vi "StateMachine.vi"() -> ()   [LabVIEW 2017]
uses:
  68b3bc89-c846-434a-a9c0-588017489639.vi
panel:
  out "number as enum":enum16{"0,01%", "0,1%", "1%", "10%", "None"}(ring)
  out "DISPLAY":string
  out "unità misura":string
  in  "num/\\":bool
  in  "num_m":bool
  in  "numK":bool
  in  "numM":bool
  in  "numC":bool
  in  "numSegn":bool
  in  "num0":bool
  in  "numVirg":bool
  in  "num9":bool
  in  "num8":bool
  in  "num7":bool
  in  "num6":bool
  in  "num5":bool
  in  "num4":bool
  in  "num2":bool
  in  "num3":bool
  in  "numEnter":bool
  in  "num1":bool
  out "displayTasterino":string
  in  "SHIFT":bool
  in  "ENTER":bool
  in  "EXIT":bool
  in  "RATE":bool
  in  "DIGITS":bool
  in  "RESTR":bool
  in  "SAVE":bool
  in  "SCAN":bool
  in  "STEP":bool
  in  "RECALL":bool
  in  "STORE":bool
  in  "ON/OFF":bool
  in  "VALUE":bool
  in  "RIGHTARR":bool
  in  "LEFTARR":bool
  in  "TRIG":bool
  in  "EX TRIG":bool
  in  "RANGE DOWN":bool
  in  "AUTO":bool
  in  "RANGE UP":bool
  out "rel":string
  out "filt":string
  out "fast 0.1 PLC":string
  out "slow 5 PLC":string
  out "auto":string
  out "med 1 PLC":string
  out "CH2":string
  out "CH1":string
  in  "TEMP 2":bool
  in  "TEMP1":bool
  in  "REL":bool
  in  "FILT":bool
  in  "ACAL":bool
  in  "V1/V2":bool
  in  "DCV2":bool
  in  "DCV1":bool
  out "shift":string
  # "MX+B"
  # "%"
  # "V1 - V2"
  # "LSYNC"
  # "TYPE"
  # "OUTPUT"
  # "AOUT"
  # "TCOUPL"
  # "RANGE"
  # "SHIFT"
  # "LIMITS"
  # "BUFFER"
  # "DELAY"
  # "HOLD"
  # "RANGE"
  # "SETUP"
  # "RS232"
  # "CONFIG"
  # "HALT"
  # "GPIB"
  # "CAL"
  # "TEST"
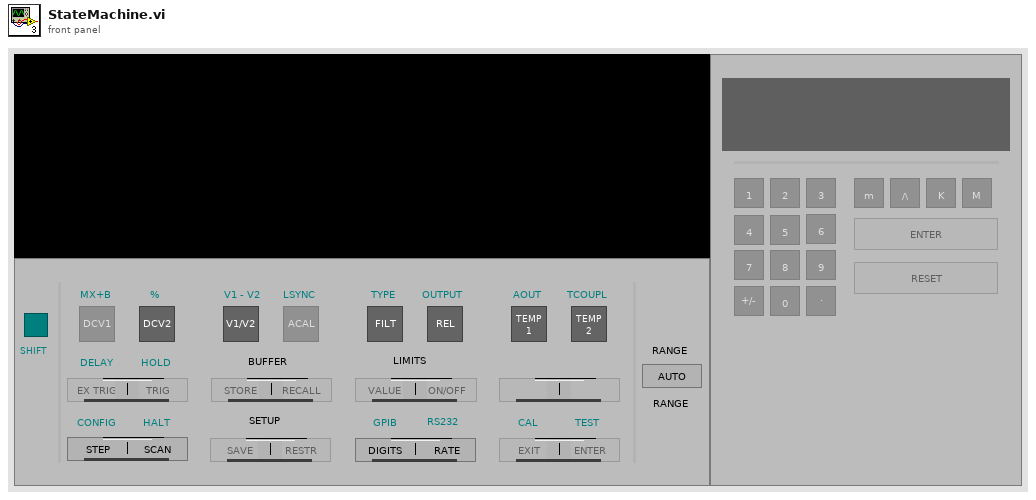
[diagram p1: front panel]
types:
  T1 = cluster{"Auto1":bool, "Auto2":bool, "Rel1":bool, "Rel2":bool, "Filt1":bool, "Filt2":bool, "Rate":enum16{"Slow", "Fast", "Med"}, "Range1":enum16{"10mV", "100mV", "1V", "10V", "100V"}, "Range2":enum16{"100mV", "1V", "10V"}, "Filt3":bool, "Filt4":bool, "Rel temp 1":bool, "Analog1":bool, "Analog2":bool, "Analog temp 1":bool, "Digital1":bool, "Digital2":bool, "Digital temp 1 ":bool, "Window1":enum16{"0,01%", "0,1%", "1%", "10%", "None"}, "Window2":enum16{"0,01%", "0,1%", "1%", "10%", "None"}, "Window temp 1":enum16{"0,01%", "0,1%", "1%", "10%", "None"}, "RDGS1":string, "RDGS2":string, "RDGS temp 1":string, "Type_type1":bool, "Type_type2":bool, "Type_type temp 1":bool, "LSync":bool, "Unit":enum16{"C", "K", "F"}, "Sens":bool, "Type tcoupl":enum16{"J", "K", "T", "E", "R", "S", "B", "N"}, "Junc":bool, "prevState":i32, "Rel temp 2":bool, "Analog temp 2":bool, "Digital temp 2":bool, "Type_type temp 2":bool, "RDGS temp 2":string, "Window temp 2":enum16{"0,01%", "0,1%", "1%", "10%", "None"}, "address":string}
  T2 = enum16{"init", "shift", "ch2", "temp1", "temp2", "v1/v2", "step", "scan", "shift_bis_volt", "v1-v2", "type_analog"}
  T3 = enum8{"Enabled", "Disabled", "Disabled and Grayed Out"}
  T4 = cluster{"Auto1":bool, "Auto2":bool, "Rel1":bool, "Rel2":bool, "Filt1":bool, "Filt2":bool, "Rate":u16, "Range1":enum16{"10mV", "100mV", "1V", "10V", "100V"}, "Range2":enum16{"100mV", "1V", "10V"}, "Filt3":bool, "Filt4":bool, "Rel temp 1":bool, "Analog1":bool, "Analog2":bool, "Analog temp 1":bool, "Digital1":bool, "Digital2":bool, "Digital temp 1 ":bool, "Window1":u16, "Window2":enum16{"0,01%", "0,1%", "1%", "10%", "None"}, "Window temp 1":enum16{"0,01%", "0,1%", "1%", "10%", "None"}, "RDGS1":string, "RDGS2":string, "RDGS temp 1":string, "Type_type1":bool, "Type_type2":bool, "Type_type temp 1":bool, "LSync":bool, "Unit":enum16{"C", "K", "F"}, "Sens":bool, "Type tcoupl":enum16{"J", "K", "T", "E", "R", "S", "B", "N"}, "Junc":bool, "prevState":i32, "Rel temp 2":bool, "Analog temp 2":bool, "Digital temp 2":bool, "Type_type temp 2":bool, "RDGS temp 2":string, "Window temp 2":enum16{"0,01%", "0,1%", "1%", "10%", "None"}, "address":string}
  T5 = cluster{"Auto1":bool, "Auto2":bool, "Rel1":bool, "Rel2":bool, "Filt1":bool, "Filt2":bool, "Rate":enum16{"Slow", "Fast", "Med"}, "Range1":enum16{"10mV", "100mV", "1V", "10V", "100V"}, "Range2":enum16{"100mV", "1V", "10V"}, "Filt3":bool, "Filt4":bool, "Rel temp 1":bool, "Analog1":bool, "Analog2":bool, "Analog temp 1":bool, "Digital1":bool, "Digital2":bool, "Digital temp 1 ":bool, "Window1":enum16{"0,01%", "0,1%", "1%", "10%", "None"}, "Window2":enum16{"0,01%", "0,1%", "1%", "10%", "None"}, "Window temp 1":enum16{"0,01%", "0,1%", "1%", "10%", "None"}, "RDGS1":string, "RDGS2":string, "RDGS temp 1":string, "Type_type1":bool, "Type_type2":bool, "Type_type temp 1":bool, "LSync":bool, "Unit":enum16{"C", "K", "F"}, "Sens":bool, "Type tcoupl":enum16{"J", "K", "T", "E", "R", "S", "B", "N"}, "Junc":bool, "prevState":i32, "Rel temp 2":bool, "Analog temp 2":bool, "Digital temp 2":bool, "Type_type temp 2":bool, "RDGS temp 2":string, "Window temp 2":enum16{"0,01%", "0,1%", "1%", "10%", "None"}, "addres":string}
  T6 = cluster{"Auto1":bool, "Auto2":bool, "Rel1":bool, "Rel2":bool, "Filt1":bool, "Filt2":bool, "Rate":enum16{"Slow", "Med", "Fast"}, "Range1":enum16{"10mV", "100mV", "1V", "10V", "100V"}, "Range2":enum16{"100mV", "1V", "10V"}, "Filt3":bool, "Filt4":bool, "Rel temp 1":bool, "Analog1":bool, "Analog2":bool, "Analog temp 1":bool, "Digital1":bool, "Digital2":bool, "Digital temp 1 ":bool, "Window1":enum16{"0,01%", "0,1%", "1%", "10%", "None"}, "Window2":enum16{"0,01%", "0,1%", "1%", "10%", "None"}, "Window temp 1":enum16{"0,01%", "0,1%", "1%", "10%", "None"}, "RDGS1":string, "RDGS2":string, "RDGS temp 1":string, "Type_type1":bool, "Type_type2":bool, "Type_type temp 1":bool, "LSync":bool, "Unit":enum16{"C", "K", "F"}, "Sens":bool, "Type tcoupl":enum16{"J", "K", "T", "E", "R", "S", "B", "N"}, "Junc":bool, "prevState":i32, "Rel temp 2":bool, "Analog temp 2":bool, "Digital temp 2":bool, "Type_type temp 2":bool, "RDGS temp 2":string, "Window temp 2":enum16{"0,01%", "0,1%", "1%", "10%", "None"}, "addres":string}
  T7 = cluster{"Auto1":bool, "Auto2":bool, "Rel1":bool, "Rel2":bool, "Filt1":bool, "Filt2":bool, "Rate":enum16{"Slow", "Med", "Fast"}, "Range1":enum16{"10mV", "100mV", "1V", "10V", "100V"}, "Range2":enum16{"100mV", "1V", "10V"}, "Filt3":bool, "Filt4":bool, "Rel temp 1":bool, "Analog1":bool, "Analog2":bool, "Analog temp 1":bool, "Digital1":bool, "Digital2":bool, "Digital temp 1 ":bool, "Window1":enum16{"0,01%", "0,1%", "1%", "10%", "None"}, "Window2":enum16{"0,01%", "0,1%", "1%", "10%", "None"}, "Window temp 1":enum16{"0,01%", "0,1%", "1%", "10%", "None"}, "RDGS1":string, "RDGS2":string, "RDGS temp 1":string, "Type_type1":bool, "Type_type2":bool, "Type_type temp 1":bool, "LSync":bool, "Unit":enum16{"C", "K", "F"}, "Sens":bool, "Type tcoupl":enum16{"J", "K", "T", "E", "R", "S", "B", "N"}, "Junc":bool, "prevState":i32, "Rel temp 2":bool, "Analog temp 2":bool, "Digital temp 2":bool, "Type_type temp 2":bool, "RDGS temp 2":string, "Window temp 2":enum16{"0,01%", "0,1%", "1%", "10%", "None"}, "address":string}
  T8 = cluster{"Auto1":bool, "Auto2":bool, "Rel1":bool, "Rel2":bool, "Filt1":bool, "Filt2":bool, "Rate":enum16{"Slow", "Fast", "Med"}, "Range1":enum16{"10mV", "100mV", "1V", "10V", "100V"}, "Range2":enum16{"100mV", "1V", "10V"}, "Filt3":bool, "Filt4":bool, "Rel temp 1":bool, "Analog1":bool, "Analog2":bool, "Analog temp 1":bool, "Digital1":bool, "Digital2":bool, "Digital temp 1 ":bool, "Window1":enum16{"None", "0,01%", "0,1%", "1%", "10%"}, "Window2":enum16{"0,01%", "0,1%", "1%", "10%", "None"}, "Window temp 1":enum16{"0,01%", "0,1%", "1%", "10%", "None"}, "RDGS1":string, "RDGS2":string, "RDGS temp 1":string, "Type_type1":bool, "Type_type2":bool, "Type_type temp 1":bool, "LSync":bool, "Unit":enum16{"C", "K", "F"}, "Sens":bool, "Type tcoupl":enum16{"J", "K", "T", "E", "R", "S", "B", "N"}, "Junc":bool, "prevState":i32, "Rel temp 2":bool, "Analog temp 2":bool, "Digital temp 2":bool, "Type_type temp 2":bool, "RDGS temp 2":string, "Window temp 2":enum16{"0,01%", "0,1%", "1%", "10%", "None"}, "address":string}
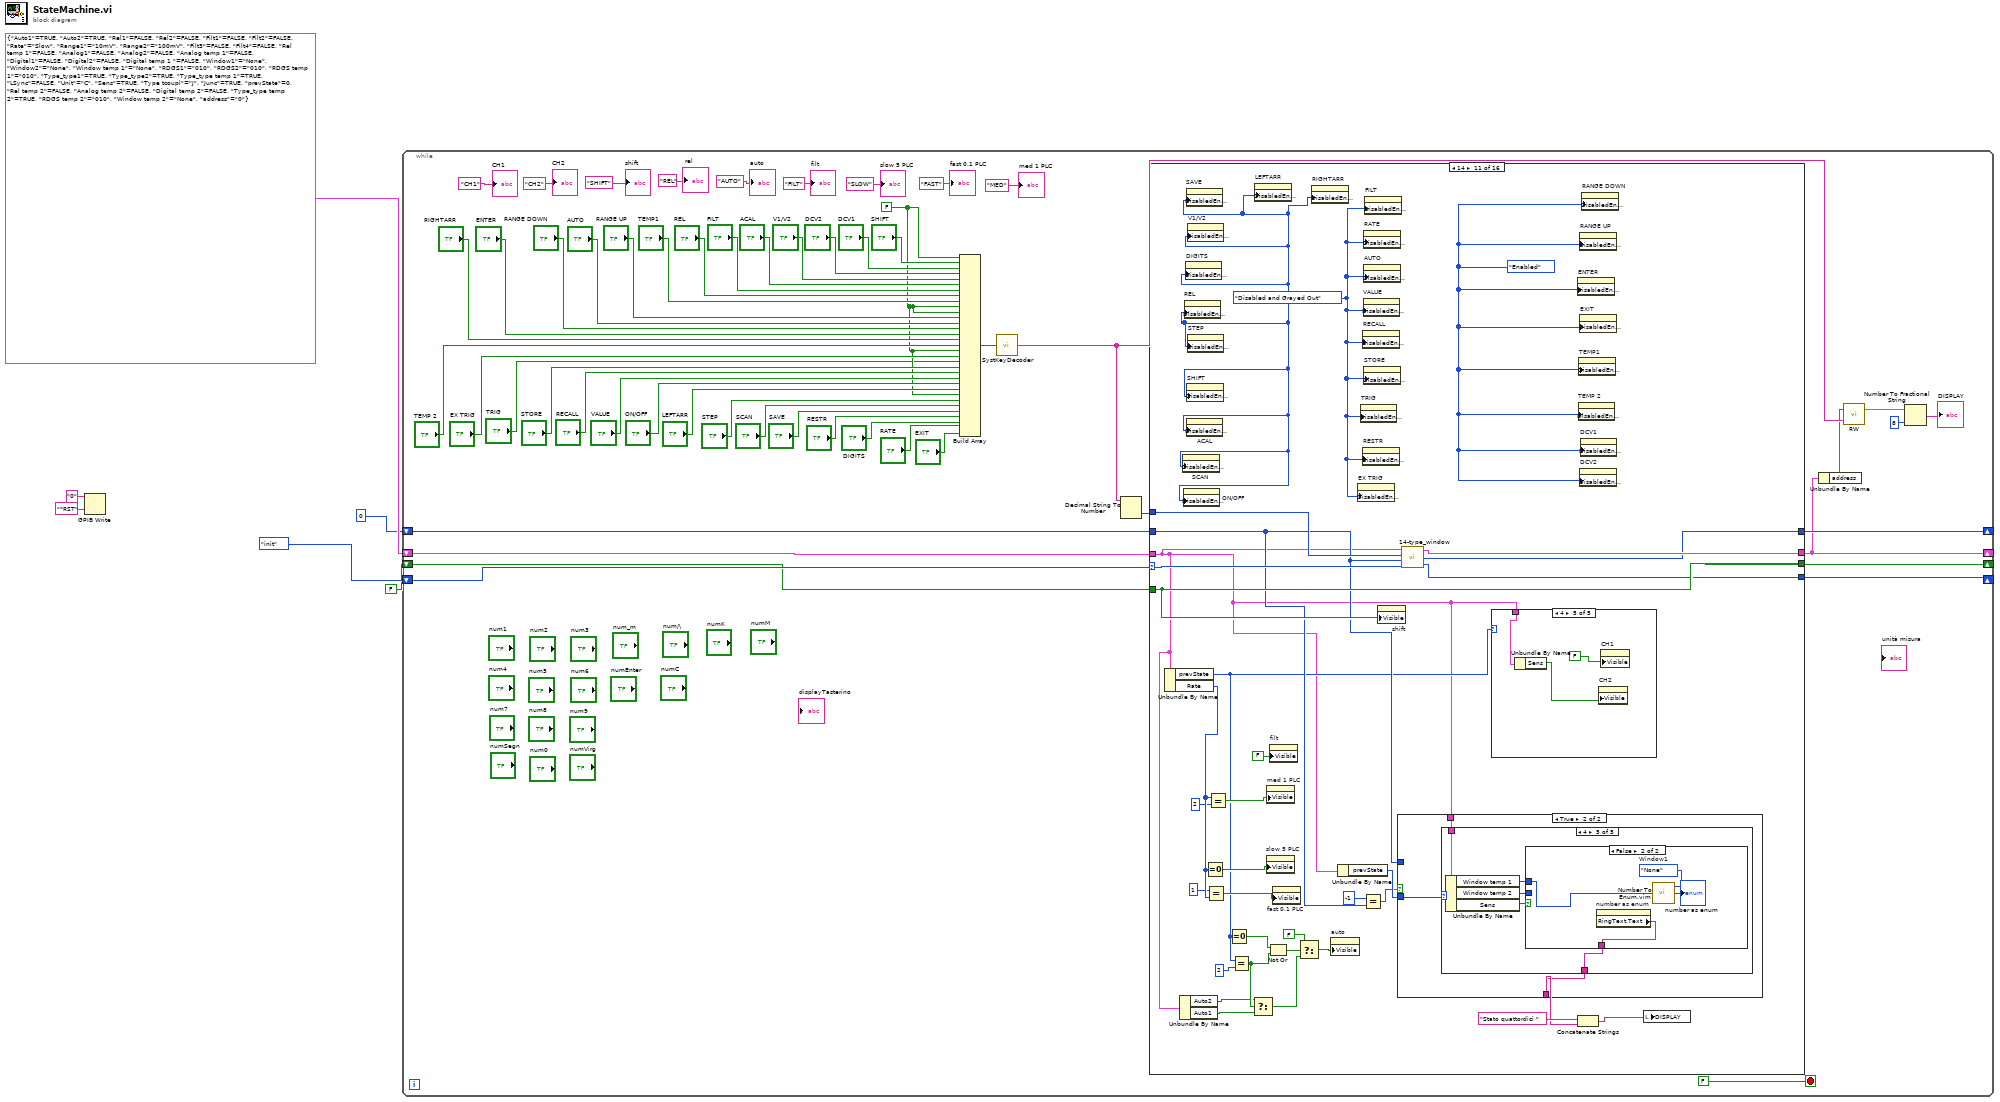
[diagram p0: block diagram]
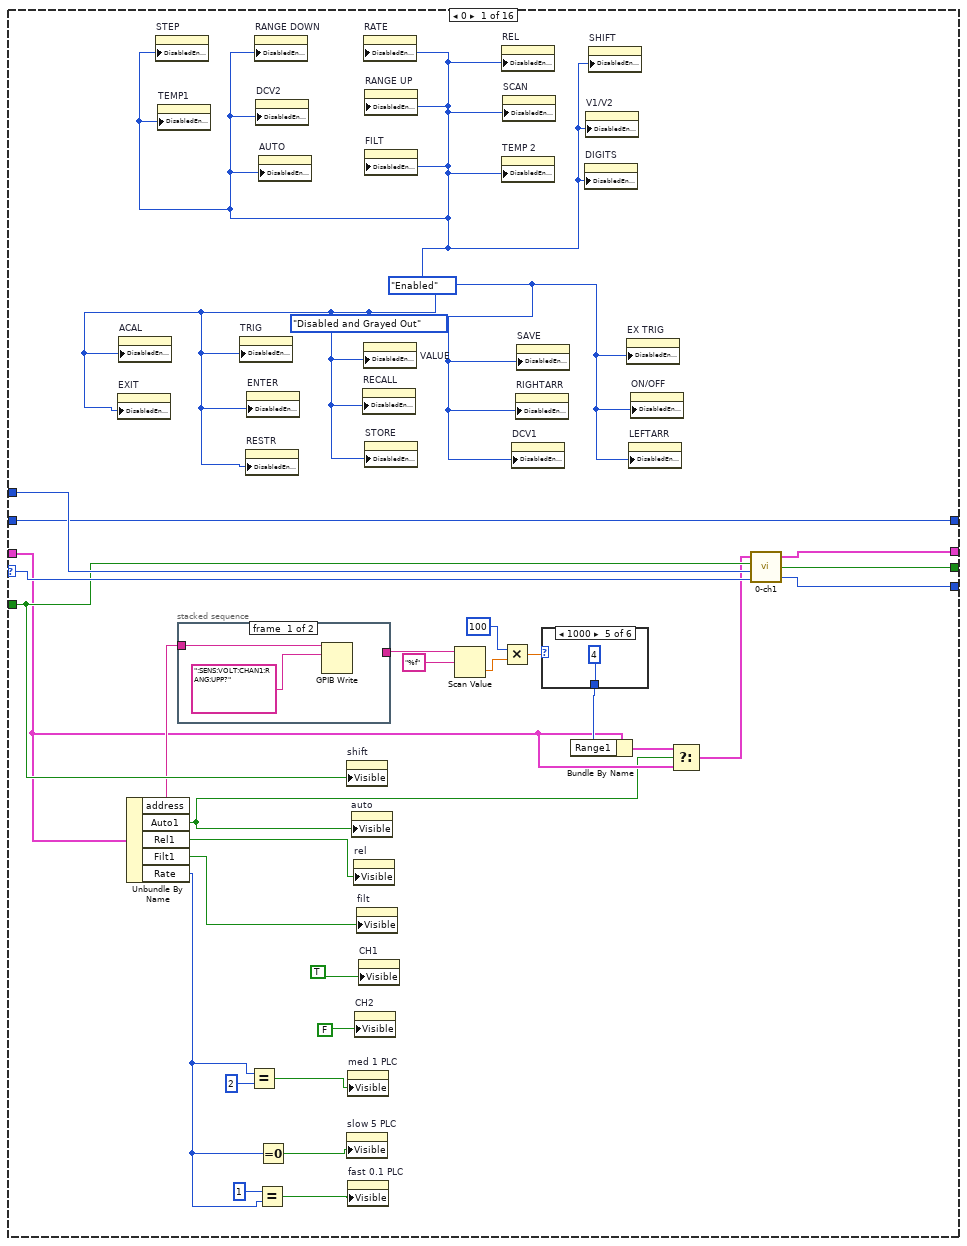
[diagram p2: hidden frame]
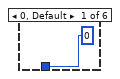
[diagram p3: hidden frame]
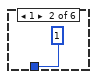
[diagram p4: hidden frame]
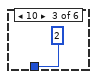
[diagram p5: hidden frame]
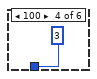
[diagram p6: hidden frame]
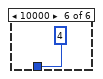
[diagram p7: hidden frame]
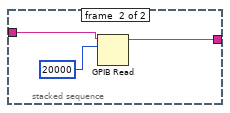
[diagram p8: hidden frame]
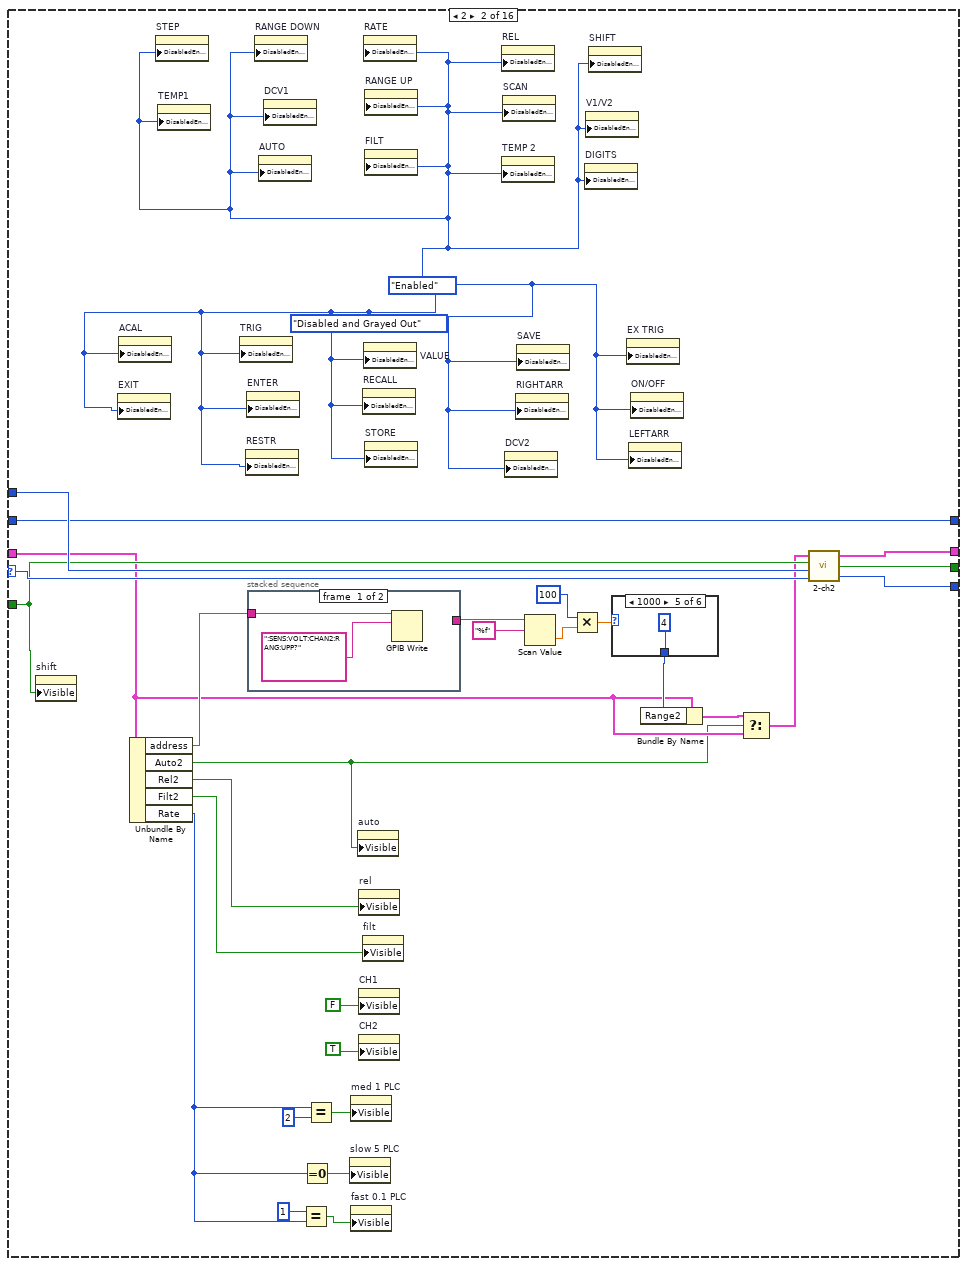
[diagram p9: hidden frame]
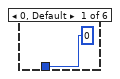
[diagram p10: hidden frame]
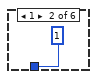
[diagram p11: hidden frame]
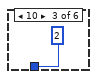
[diagram p12: hidden frame]
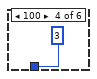
[diagram p13: hidden frame]
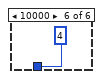
[diagram p14: hidden frame]
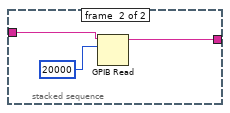
[diagram p15: hidden frame]
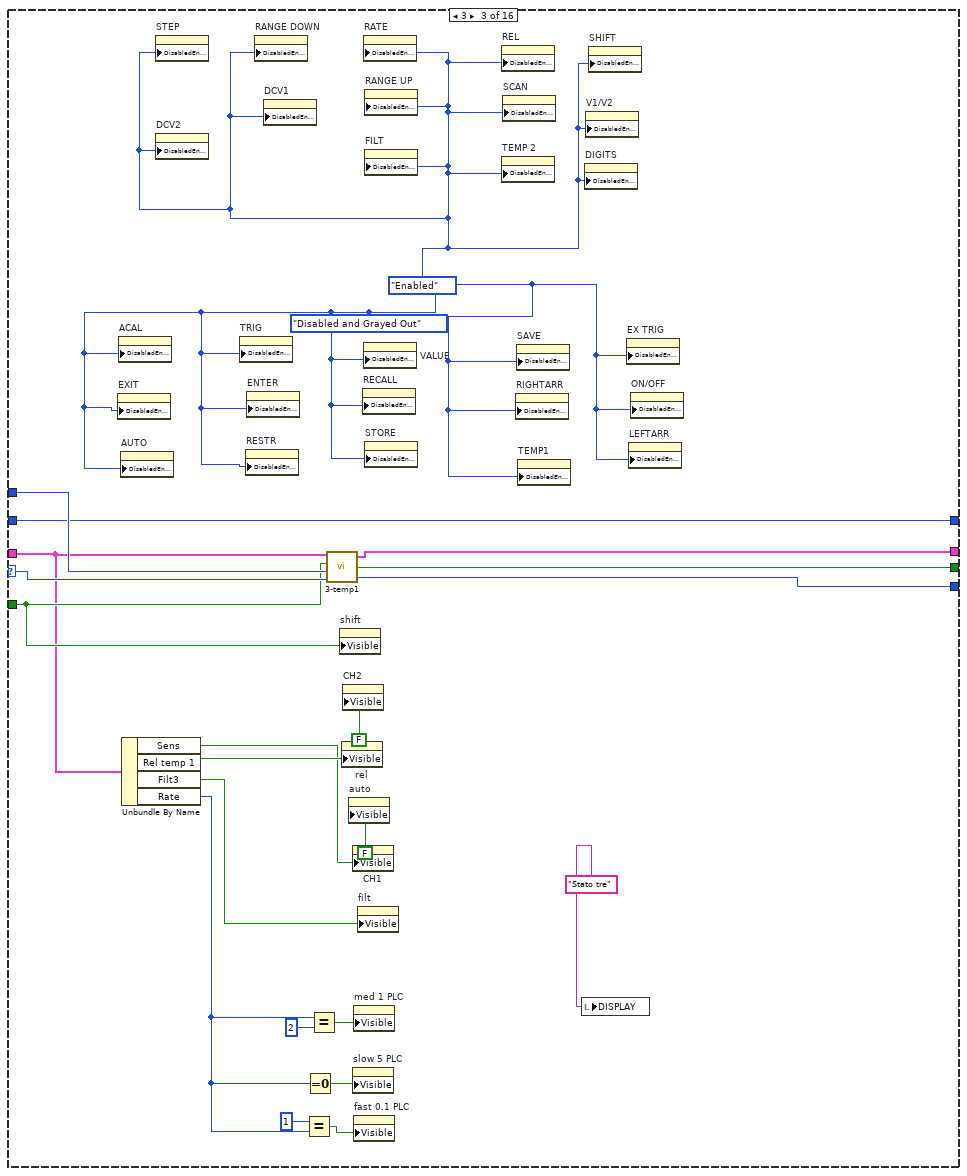
[diagram p16: hidden frame]
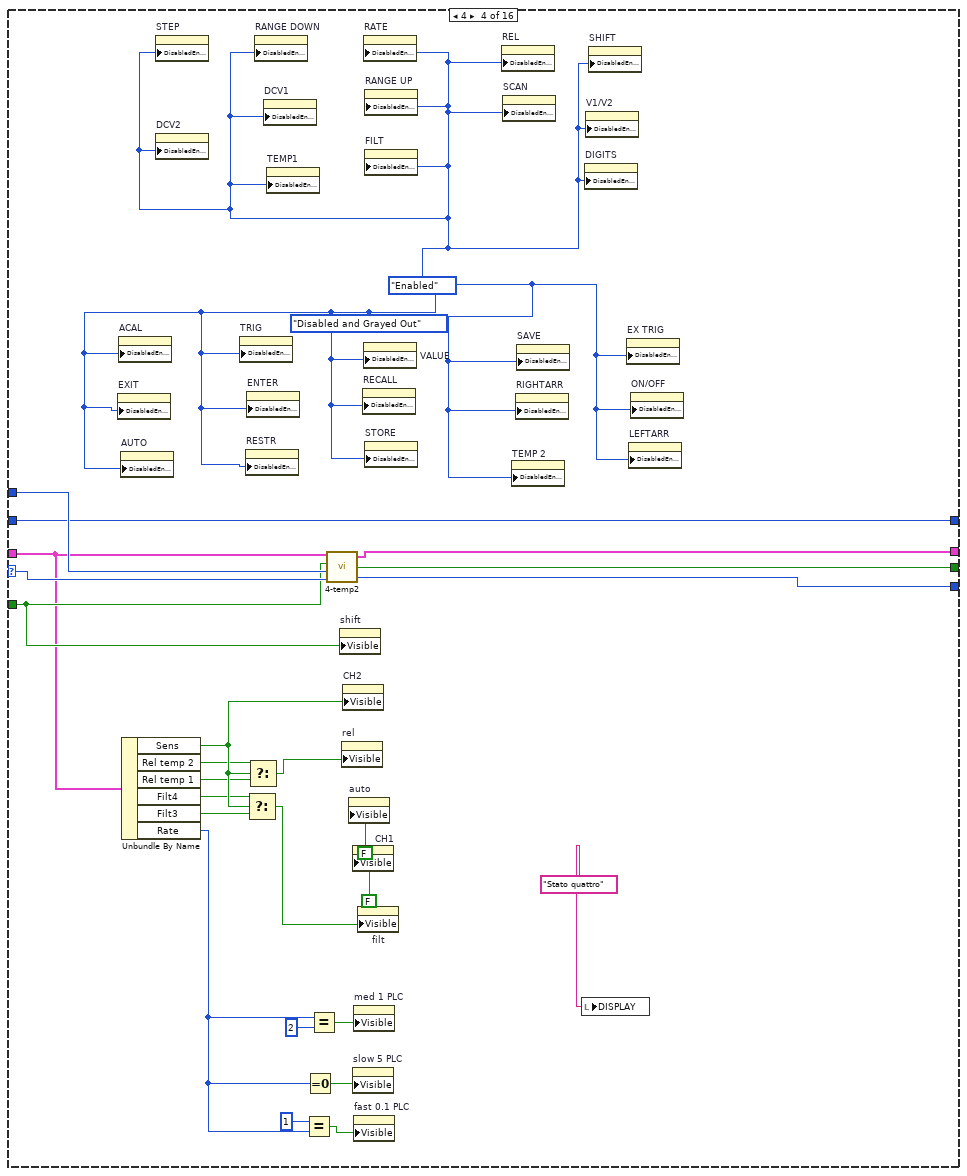
[diagram p17: hidden frame]
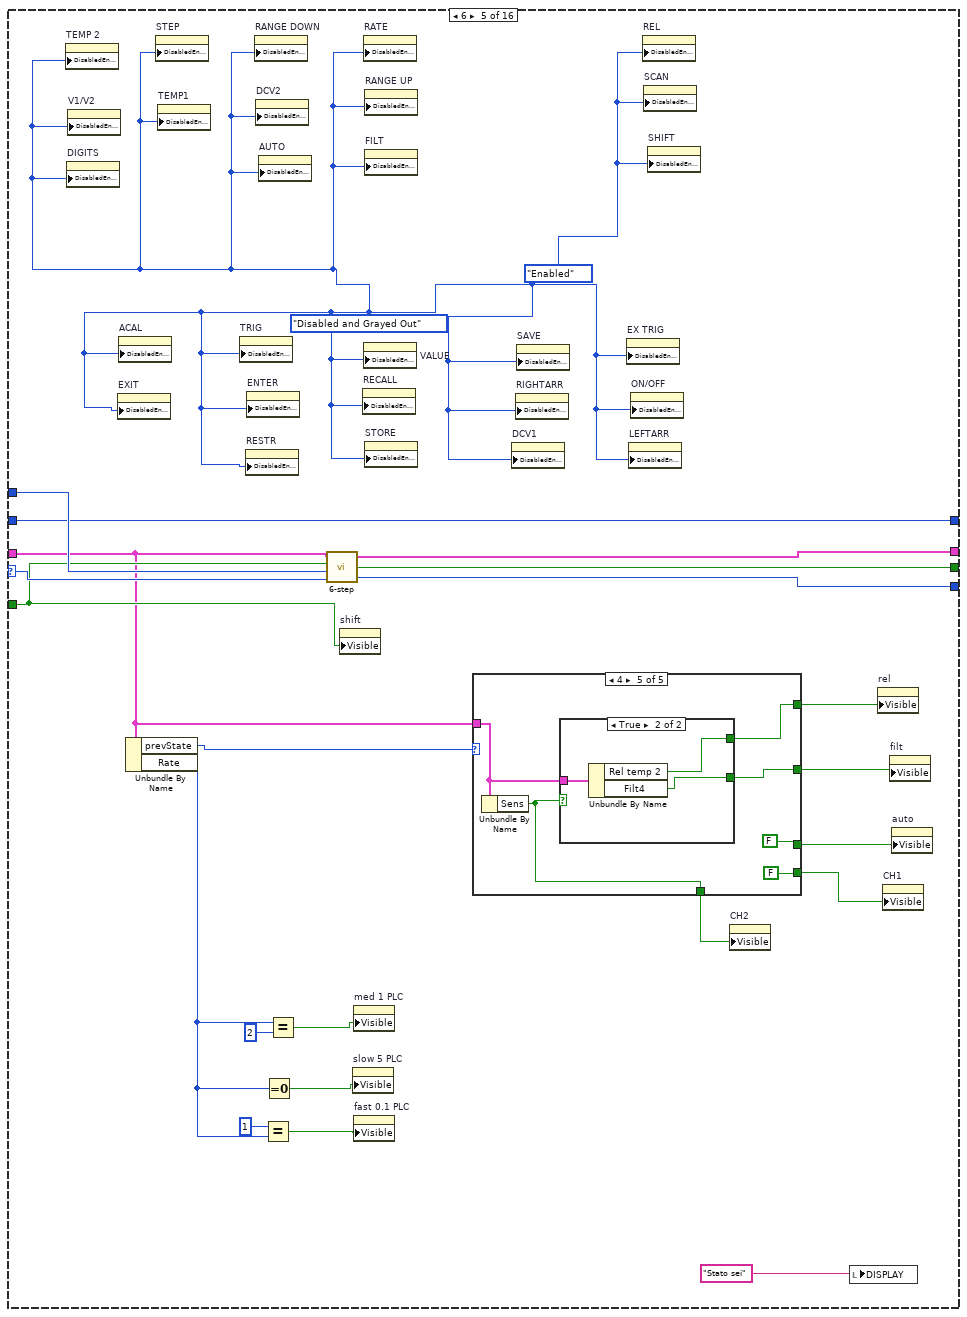
[diagram p18: hidden frame]
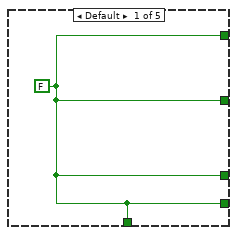
[diagram p19: hidden frame]
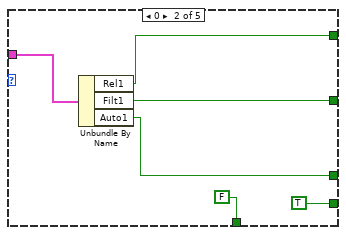
[diagram p20: hidden frame]
diagram:
  n1 = GPIB Write(0:"0" ("address string"), 1:"*RST" ("data")) -> ()  [unwired: 3 in, 2 out]
  n2 = while {
    shift-right: [w49] -> _
    shift-left: T2."init" -> [w58]
    shift-right: [w11] -> _
    shift-left: T1 {"Auto1"=TRUE, "Auto2"=TRUE, "Rel1"=FALSE, "Rel2"=FALSE, "Filt1"=FALSE, "Filt2"=FALSE, "Rate"=enum."Slow", "Range1"=enum."10mV", "Range2"=enum."100mV", "Filt3"=FALSE, "Filt4"=FALSE, "Rel temp 1"=FALSE, "Analog1"=FALSE, "Analog2"=FALSE, "Analog temp 1"=FALSE, "Digital1"=FALSE, "Digital2"=FALSE, "Digital temp 1 "=FALSE, "Window1"=enum."None", "Window2"=enum."None", "Window temp 1"=enum."None", "RDGS1"="010", "RDGS2"="010", "RDGS temp 1"="010", "Type_type1"=TRUE, "Type_type2"=TRUE, "Type_type temp 1"=TRUE, "LSync"=FALSE, "Unit"=enum."C", "Sens"=TRUE, "Type tcoupl"=enum."J", "Junc"=TRUE, "prevState"=0, "Rel temp 2"=FALSE, "Analog temp 2"=FALSE, "Digital temp 2"=FALSE, "Type_type temp 2"=TRUE, "RDGS temp 2"="010", "Window temp 2"=enum."None", "address"="0"} -> [w13]
    shift-right: [w17] -> _
    shift-left: FALSE ("shift out") -> [w16]
    shift-right: [w15] -> _
    shift-left: 0 ("Count out") -> [w14]
    stop <- FALSE stop-if-true
    w28 = FALSE
    n3 = Build Array(w28, "SHIFT", "DCV1", "DCV2", "V1/V2", "ACAL", "FILT", "REL", "TEMP1", w28, w28, "RANGE UP", "AUTO", "RANGE DOWN", "ENTER", "RIGHTARR", "TEMP 2", w28, "EX TRIG", "TRIG", "STORE", "RECALL", "VALUE", "ON/OFF", "LEFTARR", w28, "STEP", "SCAN", "SAVE", "RESTR", "DIGITS", "RATE", "EXIT") -> (w19:bool[])
    n4 = call "SystKeyDecoder.vi"("1D array"=w19) -> ("String"=w12:string)
    n5 = Decimal String To Number(string=w12) -> (number=w18:i32)  [unwired: 2 in, 1 out]
    n6 = case shown="14" w58 {
      selector: w58 -> [w90 w131 w164 w190 w213 w266 w297 w336 w415 w455 w539 w592 w627 w668 w699 w710]
      tunnel: w13 -> [w64 w105 w151 w180 w199 w250 w282 w321 w400 w436 w520 w588 w617 w664 w695 w711]
      tunnel: [w80 w123 w150 w179 w208 w258 w292 w337 w410 w456 w540 w593 w628 w669 w700 w711] -> w11
      tunnel: [w89 w130 w163 w189 w212 w265 w296 w335 w414 w454 w538 w591 w626 w667 w698 w710] -> w49
      tunnel: w18 -> [w88 w129 w162 w188 w211 w264 w298 w338 w416 w457 w541 w594 w629 w670 w701 _]
      tunnel: [w87 w128 w161 w187 w210 w263 w295 w341 w413 w460 w543 w597 w630 w671 w702 w709] -> w17
      tunnel: w16 -> [w84 w127 w160 w186 w209 w262 w295 w341 w413 w460 w543 w597 w630 w671 w702 w709]
      tunnel: [w75 w116 w145 w167 w198 w247 w291 w331 w409 w449 w533 w585 w622 -1 ("Count out") w683 w708] -> w15
      tunnel: w14 -> [w75 w116 w145 w167 w198 w247 w291 w329 w409 w447 w531 w585 w620 _ w676 w708]
      frame 0 {
        w85 = T3."Disabled and Grayed Out" ("Disabled")
        w86 = T3."Enabled" ("Disabled")
        n7 = property on="EXIT" class="Bool"("DisabledEnum"=w85) -> ()  [unwired: 2 in, 2 out]
        n8 = property on="ACAL" class="Bool"("DisabledEnum"=w85) -> ()  [unwired: 2 in, 2 out]
        n9 = Unbundle By Name(w64) -> ("address"=w65:string, "Auto1"=w62:bool, "Rel1"=w72:bool, "Filt1"=w81:bool, "Rate"=w79:u16)
        n10 = property on="STEP" class="Bool"("DisabledEnum"=w86) -> ()  [unwired: 2 in, 2 out]
        n11 = property on="TEMP1" class="Bool"("DisabledEnum"=w86) -> ()  [unwired: 2 in, 2 out]
        n12 = stacked-sequence {
          tunnel: w65 -> [w97 w100]
          tunnel: [_ w99] -> w70
          frame #0 {
            n13 = GPIB Write(0:w97, 1:":SENS:VOLT:CHAN1:RANG:UPP?" ("data")) -> ()  [unwired: 3 in, 2 out]
          }
          frame #1 {
            n14 = GPIB Read(0:w100, 1:20000 ("byte count")) -> (5:w99:string)  [unwired: 3 in, 2 out]
          }
        }
        n15 = property on="TRIG" class="Bool"("DisabledEnum"=w85) -> ()  [unwired: 2 in, 2 out]
        n16 = property on="RESTR" class="Bool"("DisabledEnum"=w85) -> ()  [unwired: 2 in, 2 out]
        n17 = property on="ENTER" class="Bool"("DisabledEnum"=w85) -> ()  [unwired: 2 in, 2 out]
        n18 = Equal?(x=w79, y=u16 2) -> (x = y?=w78:bool)
        n19 = property on="RANGE DOWN" class="Bool"("DisabledEnum"=w86) -> ()  [unwired: 2 in, 2 out]
        n20 = property on="DCV2" class="Bool"("DisabledEnum"=w86) -> ()  [unwired: 2 in, 2 out]
        n21 = Equal?(x=u16 1, y=w79) -> (x = y?=w76:bool)
        n22 = Equal To 0?(x=w79) -> (x = 0?=w77:bool)
        n23 = property on="AUTO" class="Bool"("DisabledEnum"=w86) -> ()  [unwired: 2 in, 2 out]
        n24 = property on="shift" class="Str"("Visible"=w84) -> ()  [unwired: 2 in, 2 out]
        n25 = property on="slow 5 PLC" class="Str"("Visible"=w77) -> ()  [unwired: 2 in, 2 out]
        n26 = property on="med 1 PLC" class="Str"("Visible"=w78) -> ()  [unwired: 2 in, 2 out]
        n27 = property on="fast 0.1 PLC" class="Str"("Visible"=w76) -> ()  [unwired: 2 in, 2 out]
        n28 = property on="auto" class="Str"("Visible"=w62) -> ()  [unwired: 2 in, 2 out]
        n29 = property on="rel" class="Str"("Visible"=w72) -> ()  [unwired: 2 in, 2 out]
        n30 = property on="CH2" class="Str"("Visible"=FALSE) -> ()  [unwired: 2 in, 2 out]
        n31 = property on="filt" class="Str"("Visible"=w81) -> ()  [unwired: 2 in, 2 out]
        n32 = property on="CH1" class="Str"("Visible"=TRUE) -> ()  [unwired: 2 in, 2 out]
        n33 = property on="RECALL" class="Bool"("DisabledEnum"=w85) -> ()  [unwired: 2 in, 2 out]
        n34 = property on="RATE" class="Bool"("DisabledEnum"=w86) -> ()  [unwired: 2 in, 2 out]
        n35 = property on="VALUE" class="Bool"("DisabledEnum"=w85) -> ()  [unwired: 2 in, 2 out]
        n36 = property on="RANGE UP" class="Bool"("DisabledEnum"=w86) -> ()  [unwired: 2 in, 2 out]
        n37 = property on="FILT" class="Bool"("DisabledEnum"=w86) -> ()  [unwired: 2 in, 2 out]
        n38 = property on="STORE" class="Bool"("DisabledEnum"=w85) -> ()  [unwired: 2 in, 2 out]
        n39 = Scan Value(string=w70, format string="%f") -> (value=w68:dbl)  [unwired: 1 in, 1 out]
        n40 = property on="REL" class="Bool"("DisabledEnum"=w86) -> ()  [unwired: 2 in, 2 out]
        n41 = property on="TEMP 2" class="Bool"("DisabledEnum"=w86) -> ()  [unwired: 2 in, 2 out]
        n42 = Multiply(x=100, y=w68) -> (x*y=w69:dbl)
        n43 = property on="SCAN" class="Bool"("DisabledEnum"=w86) -> ()  [unwired: 2 in, 2 out]
        n44 = property on="DCV1" class="Bool"("DisabledEnum"=w85) -> ()  [unwired: 2 in, 2 out]
        n45 = property on="RIGHTARR" class="Bool"("DisabledEnum"=w85) -> ()  [unwired: 2 in, 2 out]
        n46 = property on="SAVE" class="Bool"("DisabledEnum"=w85) -> ()  [unwired: 2 in, 2 out]
        n47 = case shown="1000" w69 {
          tunnel: [0 1 2 3 4 4] -> w71
          frame 0, Default {
          }
          frame 1 {
          }
          frame 10 {
          }
          frame 100 {
          }
          frame 1000 {
          }
          frame 10000 {
          }
        }
        n48 = Bundle By Name(cluster=w64, "Range1"=w71) -> (w63:T4)
        n49 = property on="DIGITS" class="Bool"("DisabledEnum"=w86) -> ()  [unwired: 2 in, 2 out]
        n50 = property on="V1/V2" class="Bool"("DisabledEnum"=w86) -> ()  [unwired: 2 in, 2 out]
        n51 = property on="SHIFT" class="Bool"("DisabledEnum"=w86) -> ()  [unwired: 2 in, 2 out]
        n52 = property on="EX TRIG" class="Bool"("DisabledEnum"=w85) -> ()  [unwired: 2 in, 2 out]
        n53 = property on="LEFTARR" class="Bool"("DisabledEnum"=w85) -> ()  [unwired: 2 in, 2 out]
        n54 = property on="ON/OFF" class="Bool"("DisabledEnum"=w85) -> ()  [unwired: 2 in, 2 out]
        n55 = Select(t=w63, s=w62, f=w64) -> (s? t:f=w61:T4)
        n56 = call "0-ch1.vi"("this"=w90, "button"=w88, "shift in"=w84, "setting in"=w61) -> ("next state"=w89:i32, "shift out"=w87:bool, "settings out"=w80:T5)
      }
      frame 2 {
        w121 = T3."Disabled and Grayed Out" ("Disabled")
        w122 = T3."Enabled" ("Disabled")
        n57 = property on="shift" class="Str"("Visible"=w127) -> ()  [unwired: 2 in, 2 out]
        n58 = property on="EXIT" class="Bool"("DisabledEnum"=w121) -> ()  [unwired: 2 in, 2 out]
        n59 = property on="ACAL" class="Bool"("DisabledEnum"=w121) -> ()  [unwired: 2 in, 2 out]
        n60 = Unbundle By Name(w105) -> ("address"=w106:string, "Auto2"=w102:bool, "Rel2"=w113:bool, "Filt2"=w124:bool, "Rate"=w117:u16)
        n61 = property on="STEP" class="Bool"("DisabledEnum"=w122) -> ()  [unwired: 2 in, 2 out]
        n62 = property on="TEMP1" class="Bool"("DisabledEnum"=w122) -> ()  [unwired: 2 in, 2 out]
        n63 = property on="TRIG" class="Bool"("DisabledEnum"=w121) -> ()  [unwired: 2 in, 2 out]
        n64 = property on="RESTR" class="Bool"("DisabledEnum"=w121) -> ()  [unwired: 2 in, 2 out]
        n65 = property on="ENTER" class="Bool"("DisabledEnum"=w121) -> ()  [unwired: 2 in, 2 out]
        n66 = stacked-sequence {
          tunnel: w106 -> [w138 w141]
          tunnel: [_ w140] -> w111
          frame #0 {
            n67 = GPIB Write(0:w138, 1:":SENS:VOLT:CHAN2:RANG:UPP?" ("data")) -> ()  [unwired: 3 in, 2 out]
          }
          frame #1 {
            n68 = GPIB Read(0:w141, 1:20000 ("byte count")) -> (5:w140:string)  [unwired: 3 in, 2 out]
          }
        }
        n69 = property on="RANGE DOWN" class="Bool"("DisabledEnum"=w122) -> ()  [unwired: 2 in, 2 out]
        n70 = property on="AUTO" class="Bool"("DisabledEnum"=w122) -> ()  [unwired: 2 in, 2 out]
        n71 = property on="DCV1" class="Bool"("DisabledEnum"=w122) -> ()  [unwired: 2 in, 2 out]
        n72 = Equal?(x=u16 1, y=w117) -> (x = y?=w118:bool)
        n73 = Equal To 0?(x=w117) -> (x = 0?=w120:bool)
        n74 = Equal?(x=w117, y=u16 2) -> (x = y?=w119:bool)
        n75 = property on="slow 5 PLC" class="Str"("Visible"=w120) -> ()  [unwired: 2 in, 2 out]
        n76 = property on="med 1 PLC" class="Str"("Visible"=w119) -> ()  [unwired: 2 in, 2 out]
        n77 = property on="fast 0.1 PLC" class="Str"("Visible"=w118) -> ()  [unwired: 2 in, 2 out]
        n78 = property on="auto" class="Str"("Visible"=w102) -> ()  [unwired: 2 in, 2 out]
        n79 = property on="rel" class="Str"("Visible"=w113) -> ()  [unwired: 2 in, 2 out]
        n80 = property on="CH1" class="Str"("Visible"=FALSE) -> ()  [unwired: 2 in, 2 out]
        n81 = property on="CH2" class="Str"("Visible"=TRUE) -> ()  [unwired: 2 in, 2 out]
        n82 = property on="RECALL" class="Bool"("DisabledEnum"=w121) -> ()  [unwired: 2 in, 2 out]
        n83 = property on="filt" class="Str"("Visible"=w124) -> ()  [unwired: 2 in, 2 out]
        n84 = property on="RATE" class="Bool"("DisabledEnum"=w122) -> ()  [unwired: 2 in, 2 out]
        n85 = property on="VALUE" class="Bool"("DisabledEnum"=w121) -> ()  [unwired: 2 in, 2 out]
        n86 = property on="RANGE UP" class="Bool"("DisabledEnum"=w122) -> ()  [unwired: 2 in, 2 out]
        n87 = property on="FILT" class="Bool"("DisabledEnum"=w122) -> ()  [unwired: 2 in, 2 out]
        n88 = property on="STORE" class="Bool"("DisabledEnum"=w121) -> ()  [unwired: 2 in, 2 out]
        n89 = property on="REL" class="Bool"("DisabledEnum"=w122) -> ()  [unwired: 2 in, 2 out]
        n90 = property on="TEMP 2" class="Bool"("DisabledEnum"=w122) -> ()  [unwired: 2 in, 2 out]
        n91 = property on="SCAN" class="Bool"("DisabledEnum"=w122) -> ()  [unwired: 2 in, 2 out]
        n92 = property on="DCV2" class="Bool"("DisabledEnum"=w121) -> ()  [unwired: 2 in, 2 out]
        n93 = property on="RIGHTARR" class="Bool"("DisabledEnum"=w121) -> ()  [unwired: 2 in, 2 out]
        n94 = property on="SAVE" class="Bool"("DisabledEnum"=w121) -> ()  [unwired: 2 in, 2 out]
        n95 = Scan Value(string=w111, format string="%f") -> (value=w109:dbl)  [unwired: 1 in, 1 out]
        n96 = Multiply(x=100, y=w109) -> (x*y=w110:dbl)
        n97 = property on="DIGITS" class="Bool"("DisabledEnum"=w122) -> ()  [unwired: 2 in, 2 out]
        n98 = property on="V1/V2" class="Bool"("DisabledEnum"=w122) -> ()  [unwired: 2 in, 2 out]
        n99 = property on="SHIFT" class="Bool"("DisabledEnum"=w122) -> ()  [unwired: 2 in, 2 out]
        n100 = case shown="1000" w110 {
          tunnel: [0 1 2 3 4 4] -> w112
          frame 0, Default {
          }
          frame 1 {
          }
          frame 10 {
          }
          frame 100 {
          }
          frame 1000 {
          }
          frame 10000 {
          }
        }
        n101 = property on="EX TRIG" class="Bool"("DisabledEnum"=w121) -> ()  [unwired: 2 in, 2 out]
        n102 = property on="LEFTARR" class="Bool"("DisabledEnum"=w121) -> ()  [unwired: 2 in, 2 out]
        n103 = property on="ON/OFF" class="Bool"("DisabledEnum"=w121) -> ()  [unwired: 2 in, 2 out]
        n104 = Bundle By Name(cluster=w105, "Range2"=w112) -> (w104:T4)
        n105 = Select(t=w104, s=w102, f=w105) -> (s? t:f=w103:T4)
        n106 = call "2-ch2.vi"("this"=w131, "button"=w129, "shift in"=w127, "setting in"=w103) -> ("next state"=w130:i32, "shift out"=w128:bool, "setting out"=w123:T6)
      }
      frame 3 {
        w146 = T3."Disabled and Grayed Out" ("Disabled")
        w147 = T3."Enabled" ("Disabled")
        n107 = property on="EXIT" class="Bool"("DisabledEnum"=w146) -> ()  [unwired: 2 in, 2 out]
        n108 = property on="ACAL" class="Bool"("DisabledEnum"=w146) -> ()  [unwired: 2 in, 2 out]
        n109 = property on="AUTO" class="Bool"("DisabledEnum"=w146) -> ()  [unwired: 2 in, 2 out]
        n110 = Unbundle By Name(w151) -> ("Sens"=w149:bool, "Rel temp 1"=w158:bool, "Filt3"=w157:bool, "Rate"=w152:u16)
        n111 = property on="STEP" class="Bool"("DisabledEnum"=w147) -> ()  [unwired: 2 in, 2 out]
        n112 = property on="DCV2" class="Bool"("DisabledEnum"=w147) -> ()  [unwired: 2 in, 2 out]
        n113 = property on="TRIG" class="Bool"("DisabledEnum"=w146) -> ()  [unwired: 2 in, 2 out]
        n114 = property on="RESTR" class="Bool"("DisabledEnum"=w146) -> ()  [unwired: 2 in, 2 out]
        n115 = property on="ENTER" class="Bool"("DisabledEnum"=w146) -> ()  [unwired: 2 in, 2 out]
        n116 = property on="RANGE DOWN" class="Bool"("DisabledEnum"=w147) -> ()  [unwired: 2 in, 2 out]
        n117 = property on="DCV1" class="Bool"("DisabledEnum"=w147) -> ()  [unwired: 2 in, 2 out]
        n118 = Equal?(x=u16 1, y=w152) -> (x = y?=w153:bool)
        n119 = Equal To 0?(x=w152) -> (x = 0?=w155:bool)
        n120 = Equal?(x=w152, y=u16 2) -> (x = y?=w154:bool)
        n121 = call "3-temp1.vi"("this"=w164, "button"=w162, "shift in"=w160, "setting in"=w151) -> ("next state"=w163:i32, "shift out"=w161:bool, "setting out"=w150:T6)
        n122 = property on="shift" class="Str"("Visible"=w160) -> ()  [unwired: 2 in, 2 out]
        n123 = property on="rel" class="Str"("Visible"=w158) -> ()  [unwired: 2 in, 2 out]
        n124 = property on="CH2" class="Str"("Visible"=FALSE) -> ()  [unwired: 2 in, 2 out]
        n125 = property on="auto" class="Str"("Visible"=FALSE) -> ()  [unwired: 2 in, 2 out]
        n126 = property on="CH1" class="Str"("Visible"=w149) -> ()  [unwired: 2 in, 2 out]
        n127 = property on="slow 5 PLC" class="Str"("Visible"=w155) -> ()  [unwired: 2 in, 2 out]
        n128 = property on="med 1 PLC" class="Str"("Visible"=w154) -> ()  [unwired: 2 in, 2 out]
        n129 = property on="fast 0.1 PLC" class="Str"("Visible"=w153) -> ()  [unwired: 2 in, 2 out]
        n130 = property on="filt" class="Str"("Visible"=w157) -> ()  [unwired: 2 in, 2 out]
        n131 = property on="RECALL" class="Bool"("DisabledEnum"=w146) -> ()  [unwired: 2 in, 2 out]
        n132 = property on="RATE" class="Bool"("DisabledEnum"=w147) -> ()  [unwired: 2 in, 2 out]
        n133 = property on="VALUE" class="Bool"("DisabledEnum"=w146) -> ()  [unwired: 2 in, 2 out]
        n134 = property on="RANGE UP" class="Bool"("DisabledEnum"=w147) -> ()  [unwired: 2 in, 2 out]
        n135 = property on="FILT" class="Bool"("DisabledEnum"=w147) -> ()  [unwired: 2 in, 2 out]
        n136 = property on="STORE" class="Bool"("DisabledEnum"=w146) -> ()  [unwired: 2 in, 2 out]
        n137 = property on="REL" class="Bool"("DisabledEnum"=w147) -> ()  [unwired: 2 in, 2 out]
        n138 = property on="TEMP 2" class="Bool"("DisabledEnum"=w147) -> ()  [unwired: 2 in, 2 out]
        n139 = property on="SCAN" class="Bool"("DisabledEnum"=w147) -> ()  [unwired: 2 in, 2 out]
        n140 = property on="RIGHTARR" class="Bool"("DisabledEnum"=w146) -> ()  [unwired: 2 in, 2 out]
        n141 = property on="SAVE" class="Bool"("DisabledEnum"=w146) -> ()  [unwired: 2 in, 2 out]
        n142 = property on="TEMP1" class="Bool"("DisabledEnum"=w146) -> ()  [unwired: 2 in, 2 out]
        n143 = local write "DISPLAY"("Stato tre" ("Label.Text")) -> ()
        n144 = property on="DIGITS" class="Bool"("DisabledEnum"=w147) -> ()  [unwired: 2 in, 2 out]
        n145 = property on="V1/V2" class="Bool"("DisabledEnum"=w147) -> ()  [unwired: 2 in, 2 out]
        n146 = property on="SHIFT" class="Bool"("DisabledEnum"=w147) -> ()  [unwired: 2 in, 2 out]
        n147 = property on="EX TRIG" class="Bool"("DisabledEnum"=w146) -> ()  [unwired: 2 in, 2 out]
        n148 = property on="LEFTARR" class="Bool"("DisabledEnum"=w146) -> ()  [unwired: 2 in, 2 out]
        n149 = property on="ON/OFF" class="Bool"("DisabledEnum"=w146) -> ()  [unwired: 2 in, 2 out]
      }
      frame 4 {
        w176 = T3."Disabled and Grayed Out" ("Disabled")
        w177 = T3."Enabled" ("Disabled")
        n150 = property on="EXIT" class="Bool"("DisabledEnum"=w176) -> ()  [unwired: 2 in, 2 out]
        n151 = property on="ACAL" class="Bool"("DisabledEnum"=w176) -> ()  [unwired: 2 in, 2 out]
        n152 = property on="AUTO" class="Bool"("DisabledEnum"=w176) -> ()  [unwired: 2 in, 2 out]
        n153 = Unbundle By Name(w180) -> ("Sens"=w174:bool, "Rel temp 2"=w173:bool, "Rel temp 1"=w172:bool, "Filt4"=w171:bool, "Filt3"=w170:bool, "Rate"=w181:u16)
        n154 = property on="STEP" class="Bool"("DisabledEnum"=w177) -> ()  [unwired: 2 in, 2 out]
        n155 = property on="DCV2" class="Bool"("DisabledEnum"=w177) -> ()  [unwired: 2 in, 2 out]
        n156 = property on="TRIG" class="Bool"("DisabledEnum"=w176) -> ()  [unwired: 2 in, 2 out]
        n157 = property on="RESTR" class="Bool"("DisabledEnum"=w176) -> ()  [unwired: 2 in, 2 out]
        n158 = property on="ENTER" class="Bool"("DisabledEnum"=w176) -> ()  [unwired: 2 in, 2 out]
        n159 = Select(t=w171, s=w174, f=w170) -> (s? t:f=w168:bool)
        n160 = Select(t=w173, s=w174, f=w172) -> (s? t:f=w169:bool)
        n161 = property on="RANGE DOWN" class="Bool"("DisabledEnum"=w177) -> ()  [unwired: 2 in, 2 out]
        n162 = property on="DCV1" class="Bool"("DisabledEnum"=w177) -> ()  [unwired: 2 in, 2 out]
        n163 = property on="TEMP1" class="Bool"("DisabledEnum"=w177) -> ()  [unwired: 2 in, 2 out]
        n164 = Equal?(x=u16 1, y=w181) -> (x = y?=w182:bool)
        n165 = Equal To 0?(x=w181) -> (x = 0?=w184:bool)
        n166 = Equal?(x=w181, y=u16 2) -> (x = y?=w183:bool)
        n167 = call "4-temp2.vi"("this"=w190, "button"=w188, "shift in"=w186, "setting in"=w180) -> ("next state"=w189:i32, "shift out"=w187:bool, "setting out"=w179:T6)
        n168 = property on="shift" class="Str"("Visible"=w186) -> ()  [unwired: 2 in, 2 out]
        n169 = property on="rel" class="Str"("Visible"=w169) -> ()  [unwired: 2 in, 2 out]
        n170 = property on="CH2" class="Str"("Visible"=w174) -> ()  [unwired: 2 in, 2 out]
        n171 = property on="auto" class="Str"("Visible"=FALSE) -> ()  [unwired: 2 in, 2 out]
        n172 = property on="CH1" class="Str"("Visible"=FALSE) -> ()  [unwired: 2 in, 2 out]
        n173 = property on="slow 5 PLC" class="Str"("Visible"=w184) -> ()  [unwired: 2 in, 2 out]
        n174 = property on="med 1 PLC" class="Str"("Visible"=w183) -> ()  [unwired: 2 in, 2 out]
        n175 = property on="fast 0.1 PLC" class="Str"("Visible"=w182) -> ()  [unwired: 2 in, 2 out]
        n176 = property on="filt" class="Str"("Visible"=w168) -> ()  [unwired: 2 in, 2 out]
        n177 = property on="RECALL" class="Bool"("DisabledEnum"=w176) -> ()  [unwired: 2 in, 2 out]
        n178 = property on="RATE" class="Bool"("DisabledEnum"=w177) -> ()  [unwired: 2 in, 2 out]
        n179 = property on="VALUE" class="Bool"("DisabledEnum"=w176) -> ()  [unwired: 2 in, 2 out]
        n180 = property on="RANGE UP" class="Bool"("DisabledEnum"=w177) -> ()  [unwired: 2 in, 2 out]
        n181 = property on="FILT" class="Bool"("DisabledEnum"=w177) -> ()  [unwired: 2 in, 2 out]
        n182 = property on="STORE" class="Bool"("DisabledEnum"=w176) -> ()  [unwired: 2 in, 2 out]
        n183 = property on="REL" class="Bool"("DisabledEnum"=w177) -> ()  [unwired: 2 in, 2 out]
        n184 = property on="SCAN" class="Bool"("DisabledEnum"=w177) -> ()  [unwired: 2 in, 2 out]
        n185 = property on="TEMP 2" class="Bool"("DisabledEnum"=w176) -> ()  [unwired: 2 in, 2 out]
        n186 = property on="RIGHTARR" class="Bool"("DisabledEnum"=w176) -> ()  [unwired: 2 in, 2 out]
        n187 = property on="SAVE" class="Bool"("DisabledEnum"=w176) -> ()  [unwired: 2 in, 2 out]
        n188 = local write "DISPLAY"("Stato quattro" ("Label.Text")) -> ()
        n189 = property on="DIGITS" class="Bool"("DisabledEnum"=w177) -> ()  [unwired: 2 in, 2 out]
        n190 = property on="V1/V2" class="Bool"("DisabledEnum"=w177) -> ()  [unwired: 2 in, 2 out]
        n191 = property on="SHIFT" class="Bool"("DisabledEnum"=w177) -> ()  [unwired: 2 in, 2 out]
        n192 = property on="EX TRIG" class="Bool"("DisabledEnum"=w176) -> ()  [unwired: 2 in, 2 out]
        n193 = property on="LEFTARR" class="Bool"("DisabledEnum"=w176) -> ()  [unwired: 2 in, 2 out]
        n194 = property on="ON/OFF" class="Bool"("DisabledEnum"=w176) -> ()  [unwired: 2 in, 2 out]
      }
      frame 6 {
        w201 = T3."Disabled and Grayed Out" ("Disabled")
        w202 = T3."Enabled" ("Disabled")
        n195 = property on="TEMP 2" class="Bool"("DisabledEnum"=w201) -> ()  [unwired: 2 in, 2 out]
        n196 = property on="DIGITS" class="Bool"("DisabledEnum"=w201) -> ()  [unwired: 2 in, 2 out]
        n197 = property on="V1/V2" class="Bool"("DisabledEnum"=w201) -> ()  [unwired: 2 in, 2 out]
        n198 = property on="EXIT" class="Bool"("DisabledEnum"=w201) -> ()  [unwired: 2 in, 2 out]
        n199 = property on="ACAL" class="Bool"("DisabledEnum"=w201) -> ()  [unwired: 2 in, 2 out]
        n200 = Unbundle By Name(w199) -> ("prevState"=w200:i32, "Rate"=w206:u16)
        n201 = property on="STEP" class="Bool"("DisabledEnum"=w201) -> ()  [unwired: 2 in, 2 out]
        n202 = property on="TEMP1" class="Bool"("DisabledEnum"=w201) -> ()  [unwired: 2 in, 2 out]
        n203 = property on="TRIG" class="Bool"("DisabledEnum"=w201) -> ()  [unwired: 2 in, 2 out]
        n204 = property on="RESTR" class="Bool"("DisabledEnum"=w201) -> ()  [unwired: 2 in, 2 out]
        n205 = property on="ENTER" class="Bool"("DisabledEnum"=w201) -> ()  [unwired: 2 in, 2 out]
        n206 = property on="RANGE DOWN" class="Bool"("DisabledEnum"=w201) -> ()  [unwired: 2 in, 2 out]
        n207 = property on="DCV2" class="Bool"("DisabledEnum"=w201) -> ()  [unwired: 2 in, 2 out]
        n208 = property on="AUTO" class="Bool"("DisabledEnum"=w201) -> ()  [unwired: 2 in, 2 out]
        n209 = Equal?(x=u16 1, y=w206) -> (x = y?=w203:bool)
        n210 = Equal To 0?(x=w206) -> (x = 0?=w204:bool)
        n211 = Equal?(x=w206, y=u16 2) -> (x = y?=w205:bool)
        n212 = call "6-step.vi"("this"=w213, "button"=w211, "shift in"=w209, "settings in"=w199) -> ("next state"=w212:i32, "shift out"=w210:bool, "settings out"=w208:T6)
        n213 = property on="shift" class="Str"("Visible"=w209) -> ()  [unwired: 2 in, 2 out]
        n214 = property on="slow 5 PLC" class="Str"("Visible"=w204) -> ()  [unwired: 2 in, 2 out]
        n215 = property on="med 1 PLC" class="Str"("Visible"=w205) -> ()  [unwired: 2 in, 2 out]
        n216 = property on="fast 0.1 PLC" class="Str"("Visible"=w203) -> ()  [unwired: 2 in, 2 out]
        n217 = property on="RECALL" class="Bool"("DisabledEnum"=w201) -> ()  [unwired: 2 in, 2 out]
        n218 = property on="RATE" class="Bool"("DisabledEnum"=w201) -> ()  [unwired: 2 in, 2 out]
        n219 = property on="VALUE" class="Bool"("DisabledEnum"=w201) -> ()  [unwired: 2 in, 2 out]
        n220 = property on="RANGE UP" class="Bool"("DisabledEnum"=w201) -> ()  [unwired: 2 in, 2 out]
        n221 = property on="FILT" class="Bool"("DisabledEnum"=w201) -> ()  [unwired: 2 in, 2 out]
        n222 = property on="STORE" class="Bool"("DisabledEnum"=w201) -> ()  [unwired: 2 in, 2 out]
        n223 = case shown="4" w200 {
          tunnel: w199 -> [_ w220 w226 w232 w236]
          tunnel: [w214 w219 w223 w231 w238] -> w195
          tunnel: [w214 w218 w222 w230 w237] -> w194
          tunnel: [w214 w217 w221 FALSE ("Visible") FALSE ("Visible")] -> w193
          tunnel: [w214 TRUE ("Visible") FALSE ("Visible") w228 FALSE ("Visible")] -> w192
          tunnel: [w214 FALSE ("Visible") TRUE ("Visible") FALSE ("Visible") w235] -> w191
          frame Default {
            w214 = FALSE ("Visible")
          }
          frame 0 {
            n224 = Unbundle By Name(w220) -> ("Rel1"=w219:bool, "Filt1"=w218:bool, "Auto1"=w217:bool)
          }
          frame 2 {
            n225 = Unbundle By Name(w226) -> ("Rel2"=w223:bool, "Filt2"=w222:bool, "Auto2"=w221:bool)
          }
          frame 3 {
            n226 = Unbundle By Name(w232) -> ("Rel temp 1"=w231:bool, "Filt3"=w230:bool, "Sens"=w228:bool)
          }
          frame 4 {
            n227 = Unbundle By Name(w236) -> ("Sens"=w235:bool)
            n228 = case shown="True" w235 {
              tunnel: [w240 w244] -> w238
              tunnel: [w239 w243] -> w237
              tunnel: w236 -> [w241 w242]
              frame False {
                n229 = Unbundle By Name(w241) -> ("Rel temp 1"=w240:bool, "Filt3"=w239:bool)
              }
              frame True {
                n230 = Unbundle By Name(w242) -> ("Rel temp 2"=w244:bool, "Filt4"=w243:bool)
              }
            }
          }
        }
        n231 = property on="DCV1" class="Bool"("DisabledEnum"=w201) -> ()  [unwired: 2 in, 2 out]
        n232 = property on="RIGHTARR" class="Bool"("DisabledEnum"=w201) -> ()  [unwired: 2 in, 2 out]
        n233 = property on="SAVE" class="Bool"("DisabledEnum"=w201) -> ()  [unwired: 2 in, 2 out]
        n234 = property on="EX TRIG" class="Bool"("DisabledEnum"=w201) -> ()  [unwired: 2 in, 2 out]
        n235 = property on="LEFTARR" class="Bool"("DisabledEnum"=w201) -> ()  [unwired: 2 in, 2 out]
        n236 = property on="ON/OFF" class="Bool"("DisabledEnum"=w201) -> ()  [unwired: 2 in, 2 out]
        n237 = property on="REL" class="Bool"("DisabledEnum"=w202) -> ()  [unwired: 2 in, 2 out]
        n238 = property on="SCAN" class="Bool"("DisabledEnum"=w202) -> ()  [unwired: 2 in, 2 out]
        n239 = property on="SHIFT" class="Bool"("DisabledEnum"=w202) -> ()  [unwired: 2 in, 2 out]
        n240 = property on="CH2" class="Str"("Visible"=w191) -> ()  [unwired: 2 in, 2 out]
        n241 = local write "DISPLAY"("Stato sei" ("Label.Text")) -> ()
        n242 = property on="rel" class="Str"("Visible"=w195) -> ()  [unwired: 2 in, 2 out]
        n243 = property on="CH1" class="Str"("Visible"=w192) -> ()  [unwired: 2 in, 2 out]
        n244 = property on="filt" class="Str"("Visible"=w194) -> ()  [unwired: 2 in, 2 out]
        n245 = property on="auto" class="Str"("Visible"=w193) -> ()  [unwired: 2 in, 2 out]
      }
      frame 7 {
        w249 = T3."Disabled and Grayed Out" ("Disabled")
        w248 = T3."Enabled" ("Disabled")
        n246 = property on="TEMP 2" class="Bool"("DisabledEnum"=w249) -> ()  [unwired: 2 in, 2 out]
        n247 = property on="DIGITS" class="Bool"("DisabledEnum"=w249) -> ()  [unwired: 2 in, 2 out]
        n248 = property on="V1/V2" class="Bool"("DisabledEnum"=w249) -> ()  [unwired: 2 in, 2 out]
        n249 = property on="EXIT" class="Bool"("DisabledEnum"=w249) -> ()  [unwired: 2 in, 2 out]
        n250 = property on="ACAL" class="Bool"("DisabledEnum"=w249) -> ()  [unwired: 2 in, 2 out]
        n251 = Unbundle By Name(w250) -> ("prevState"=w251:i32, "Auto1"=w260:bool, "Rate"=w256:u16)  [unwired: 1 out]
        n252 = property on="TEMP1" class="Bool"("DisabledEnum"=w249) -> ()  [unwired: 2 in, 2 out]
        n253 = property on="TRIG" class="Bool"("DisabledEnum"=w249) -> ()  [unwired: 2 in, 2 out]
        n254 = property on="RESTR" class="Bool"("DisabledEnum"=w249) -> ()  [unwired: 2 in, 2 out]
        n255 = property on="ENTER" class="Bool"("DisabledEnum"=w249) -> ()  [unwired: 2 in, 2 out]
        n256 = property on="RANGE DOWN" class="Bool"("DisabledEnum"=w249) -> ()  [unwired: 2 in, 2 out]
        n257 = property on="DCV2" class="Bool"("DisabledEnum"=w249) -> ()  [unwired: 2 in, 2 out]
        n258 = property on="AUTO" class="Bool"("DisabledEnum"=w249) -> ()  [unwired: 2 in, 2 out]
        n259 = Equal?(x=u16 1, y=w256) -> (x = y?=w253:bool)
        n260 = Equal To 0?(x=w256) -> (x = 0?=w254:bool)
        n261 = Equal?(x=w256, y=u16 2) -> (x = y?=w255:bool)
        n262 = call "7-scan.vi"("this"=w266, "button"=w264, "shift in"=w262, "settings in"=w250) -> ("next state"=w265:i32, "shift out"=w263:bool, "settings out"=w258:T6)
        n263 = property on="shift" class="Str"("Visible"=w262) -> ()  [unwired: 2 in, 2 out]
        n264 = property on="CH2" class="Str"("Visible"=FALSE) -> ()  [unwired: 2 in, 2 out]
        n265 = property on="auto" class="Str"("Visible"=w260) -> ()  [unwired: 2 in, 2 out]
        n266 = property on="CH1" class="Str"("Visible"=TRUE) -> ()  [unwired: 2 in, 2 out]
        n267 = property on="slow 5 PLC" class="Str"("Visible"=w254) -> ()  [unwired: 2 in, 2 out]
        n268 = property on="med 1 PLC" class="Str"("Visible"=w255) -> ()  [unwired: 2 in, 2 out]
        n269 = property on="fast 0.1 PLC" class="Str"("Visible"=w253) -> ()  [unwired: 2 in, 2 out]
        n270 = property on="filt" class="Str"("Visible"=FALSE) -> ()  [unwired: 2 in, 2 out]
        n271 = property on="RECALL" class="Bool"("DisabledEnum"=w249) -> ()  [unwired: 2 in, 2 out]
        n272 = property on="RATE" class="Bool"("DisabledEnum"=w249) -> ()  [unwired: 2 in, 2 out]
        n273 = property on="VALUE" class="Bool"("DisabledEnum"=w249) -> ()  [unwired: 2 in, 2 out]
        n274 = property on="RANGE UP" class="Bool"("DisabledEnum"=w249) -> ()  [unwired: 2 in, 2 out]
        n275 = property on="FILT" class="Bool"("DisabledEnum"=w249) -> ()  [unwired: 2 in, 2 out]
        n276 = property on="STORE" class="Bool"("DisabledEnum"=w249) -> ()  [unwired: 2 in, 2 out]
        n277 = case shown="4" w251 {
          tunnel: w250 -> [_ w268 w270 w272 w277]
          frame Default {
          }
          frame 0 {
            n278 = Unbundle By Name(w268) -> ("Rel1"=w267:bool)
            n279 = property on="rel" class="Str"("Visible"=w267) -> ()  [unwired: 2 in, 2 out]
          }
          frame 2 {
            n280 = Unbundle By Name(w270) -> ("Rel2"=w269:bool)
            n281 = property on="rel" class="Str"("Visible"=w269) -> ()  [unwired: 2 in, 2 out]
          }
          frame 3 {
            n282 = Unbundle By Name(w272) -> ("Rel temp 1"=w271:bool)
            n283 = property on="rel" class="Str"("Visible"=w271) -> ()  [unwired: 2 in, 2 out]
          }
          frame 4 {
            n284 = Unbundle By Name(w277) -> ("Rel temp 2"=w275:bool, "Sens"=w276:bool, "Rel temp 1"=w274:bool)
            n285 = Select(t=w275, s=w276, f=w274) -> (s? t:f=w273:bool)
            n286 = property on="rel" class="Str"("Visible"=w273) -> ()  [unwired: 2 in, 2 out]
          }
        }
        n287 = property on="DCV1" class="Bool"("DisabledEnum"=w249) -> ()  [unwired: 2 in, 2 out]
        n288 = property on="RIGHTARR" class="Bool"("DisabledEnum"=w249) -> ()  [unwired: 2 in, 2 out]
        n289 = property on="SAVE" class="Bool"("DisabledEnum"=w249) -> ()  [unwired: 2 in, 2 out]
        n290 = local write "DISPLAY"("Stato sette" ("Label.Text")) -> ()
        n291 = property on="EX TRIG" class="Bool"("DisabledEnum"=w249) -> ()  [unwired: 2 in, 2 out]
        n292 = property on="LEFTARR" class="Bool"("DisabledEnum"=w249) -> ()  [unwired: 2 in, 2 out]
        n293 = property on="ON/OFF" class="Bool"("DisabledEnum"=w249) -> ()  [unwired: 2 in, 2 out]
        n294 = property on="REL" class="Bool"("DisabledEnum"=w248) -> ()  [unwired: 2 in, 2 out]
        n295 = property on="STEP" class="Bool"("DisabledEnum"=w248) -> ()  [unwired: 2 in, 2 out]
        n296 = property on="SHIFT" class="Bool"("DisabledEnum"=w248) -> ()  [unwired: 2 in, 2 out]
        n297 = property on="SCAN" class="Bool"("DisabledEnum"=w248) -> ()  [unwired: 2 in, 2 out]
      }
      frame 10 {
        w293 = T3."Disabled and Grayed Out" ("Disabled")
        w294 = T3."Enabled" ("Disabled")
        n298 = property on="SCAN" class="Bool"("DisabledEnum"=w293) -> ()  [unwired: 2 in, 2 out]
        n299 = property on="ON/OFF" class="Bool"("DisabledEnum"=w293) -> ()  [unwired: 2 in, 2 out]
        n300 = property on="REL" class="Bool"("DisabledEnum"=w293) -> ()  [unwired: 2 in, 2 out]
        n301 = property on="DIGITS" class="Bool"("DisabledEnum"=w293) -> ()  [unwired: 2 in, 2 out]
        n302 = property on="SAVE" class="Bool"("DisabledEnum"=w293) -> ()  [unwired: 2 in, 2 out]
        n303 = property on="ACAL" class="Bool"("DisabledEnum"=w293) -> ()  [unwired: 2 in, 2 out]
        n304 = property on="SHIFT" class="Bool"("DisabledEnum"=w293) -> ()  [unwired: 2 in, 2 out]
        n305 = property on="V1/V2" class="Bool"("DisabledEnum"=w293) -> ()  [unwired: 2 in, 2 out]
        n306 = property on="STEP" class="Bool"("DisabledEnum"=w293) -> ()  [unwired: 2 in, 2 out]
        n307 = Unbundle By Name(w282) -> ("prevState"=w281:i32, "Rate"=w303:u16)
        n308 = Equal To 0?(x=w303) -> (x = 0?=w301:bool)
        n309 = Equal?(x=u16 1, y=w303) -> (x = y?=w300:bool)
        n310 = Equal?(x=w303, y=u16 2) -> (x = y?=w302:bool)
        n311 = property on="EX TRIG" class="Bool"("DisabledEnum"=w293) -> ()  [unwired: 2 in, 2 out]
        n312 = property on="TRIG" class="Bool"("DisabledEnum"=w293) -> ()  [unwired: 2 in, 2 out]
        n313 = property on="RECALL" class="Bool"("DisabledEnum"=w293) -> ()  [unwired: 2 in, 2 out]
        n314 = property on="RESTR" class="Bool"("DisabledEnum"=w293) -> ()  [unwired: 2 in, 2 out]
        n315 = property on="VALUE" class="Bool"("DisabledEnum"=w293) -> ()  [unwired: 2 in, 2 out]
        n316 = property on="RATE" class="Bool"("DisabledEnum"=w293) -> ()  [unwired: 2 in, 2 out]
        n317 = property on="AUTO" class="Bool"("DisabledEnum"=w293) -> ()  [unwired: 2 in, 2 out]
        n318 = property on="STORE" class="Bool"("DisabledEnum"=w293) -> ()  [unwired: 2 in, 2 out]
        n319 = property on="FILT" class="Bool"("DisabledEnum"=w293) -> ()  [unwired: 2 in, 2 out]
        n320 = property on="shift" class="Str"("Visible"=w295) -> ()  [unwired: 2 in, 2 out]
        n321 = property on="slow 5 PLC" class="Str"("Visible"=w301) -> ()  [unwired: 2 in, 2 out]
        n322 = property on="med 1 PLC" class="Str"("Visible"=w302) -> ()  [unwired: 2 in, 2 out]
        n323 = property on="fast 0.1 PLC" class="Str"("Visible"=w300) -> ()  [unwired: 2 in, 2 out]
        n324 = property on="filt" class="Str"("Visible"=FALSE) -> ()  [unwired: 2 in, 2 out]
        n325 = call "10-type_analog.vi"("this"=w297, "button"=w298, "Cluster"=w282) -> ("next state"=w296:i32, "Cluster 2"=w292:T7)
        n326 = Unbundle By Name(w282) -> ("Auto2"=w285:bool, "Auto1"=w284:bool)
        n327 = Equal To 0?(x=w281) -> (x = 0?=w289:bool)
        n328 = Equal?(x=w281, y=2) -> (x = y?=w286:bool)
        n329 = case shown="0" w281 {
          tunnel: w282 -> [_ _ _ w309 w312]
          frame Default {
          }
          frame 0 {
            n330 = property on="CH1" class="Str"("Visible"=TRUE) -> ()  [unwired: 2 in, 2 out]
            n331 = property on="CH2" class="Str"("Visible"=FALSE) -> ()  [unwired: 2 in, 2 out]
          }
          frame 2 {
            n332 = property on="CH1" class="Str"("Visible"=FALSE) -> ()  [unwired: 2 in, 2 out]
            n333 = property on="CH2" class="Str"("Visible"=TRUE) -> ()  [unwired: 2 in, 2 out]
          }
          frame 3 {
            n334 = Unbundle By Name(w309) -> ("Sens"=w311:bool)
            n335 = property on="CH2" class="Str"("Visible"=FALSE) -> ()  [unwired: 2 in, 2 out]
            n336 = property on="CH1" class="Str"("Visible"=w311) -> ()  [unwired: 2 in, 2 out]
          }
          frame 4 {
            n337 = Unbundle By Name(w312) -> ("Sens"=w313:bool)
            n338 = property on="CH2" class="Str"("Visible"=w313) -> ()  [unwired: 2 in, 2 out]
            n339 = property on="CH1" class="Str"("Visible"=FALSE) -> ()  [unwired: 2 in, 2 out]
          }
        }
        n340 = Select(t=w285, s=w286, f=w284) -> (s? t:f=w283:bool)
        n341 = Not Or(1:w286, 2:w289) -> (0:w288:bool)
        n342 = Select(t=FALSE, s=w288, f=w283) -> (s? t:f=w280:bool)
        n343 = property on="auto" class="Str"("Visible"=w280) -> ()  [unwired: 2 in, 2 out]
        n344 = property on="RIGHTARR" class="Bool"("DisabledEnum"=w294) -> ()  [unwired: 2 in, 2 out]
        n345 = property on="ENTER" class="Bool"("DisabledEnum"=w294) -> ()  [unwired: 2 in, 2 out]
        n346 = property on="RANGE UP" class="Bool"("DisabledEnum"=w294) -> ()  [unwired: 2 in, 2 out]
        n347 = property on="TEMP 2" class="Bool"("DisabledEnum"=w294) -> ()  [unwired: 2 in, 2 out]
        n348 = property on="TEMP1" class="Bool"("DisabledEnum"=w294) -> ()  [unwired: 2 in, 2 out]
        n349 = property on="LEFTARR" class="Bool"("DisabledEnum"=w294) -> ()  [unwired: 2 in, 2 out]
        n350 = property on="EXIT" class="Bool"("DisabledEnum"=w294) -> ()  [unwired: 2 in, 2 out]
        n351 = property on="DCV2" class="Bool"("DisabledEnum"=w294) -> ()  [unwired: 2 in, 2 out]
        n352 = property on="RANGE DOWN" class="Bool"("DisabledEnum"=w294) -> ()  [unwired: 2 in, 2 out]
        n353 = property on="DCV1" class="Bool"("DisabledEnum"=w294) -> ()  [unwired: 2 in, 2 out]
        n354 = local write "DISPLAY"("Stato dieci" ("Label.Text")) -> ()
      }
      frame 11 {
        w339 = T3."Disabled and Grayed Out" ("Disabled")
        w340 = T3."Enabled" ("Disabled")
        n355 = Unbundle By Name(w321) -> ("prevState"=w327:i32, "Rate"=w322:u16)
        n356 = property on="SCAN" class="Bool"("DisabledEnum"=w339) -> ()  [unwired: 2 in, 2 out]
        n357 = property on="ON/OFF" class="Bool"("DisabledEnum"=w339) -> ()  [unwired: 2 in, 2 out]
        n358 = property on="REL" class="Bool"("DisabledEnum"=w339) -> ()  [unwired: 2 in, 2 out]
        n359 = property on="DIGITS" class="Bool"("DisabledEnum"=w339) -> ()  [unwired: 2 in, 2 out]
        n360 = property on="SAVE" class="Bool"("DisabledEnum"=w339) -> ()  [unwired: 2 in, 2 out]
        n361 = property on="ACAL" class="Bool"("DisabledEnum"=w339) -> ()  [unwired: 2 in, 2 out]
        n362 = property on="SHIFT" class="Bool"("DisabledEnum"=w339) -> ()  [unwired: 2 in, 2 out]
        n363 = property on="V1/V2" class="Bool"("DisabledEnum"=w339) -> ()  [unwired: 2 in, 2 out]
        n364 = property on="STEP" class="Bool"("DisabledEnum"=w339) -> ()  [unwired: 2 in, 2 out]
        n365 = Unbundle By Name(w321) -> ("Auto2"=w319:bool, "Auto1"=w318:bool)
        n366 = Equal To 0?(x=w322) -> (x = 0?=w344:bool)
        n367 = Equal?(x=u16 1, y=w322) -> (x = y?=w343:bool)
        n368 = Equal?(x=w322, y=u16 2) -> (x = y?=w345:bool)
        n369 = Equal To 0?(x=w327) -> (x = 0?=w326:bool)
        n370 = Equal?(x=w327, y=2) -> (x = y?=w320:bool)
        n371 = property on="slow 5 PLC" class="Str"("Visible"=w344) -> ()  [unwired: 2 in, 2 out]
        n372 = Select(t=w319, s=w320, f=w318) -> (s? t:f=w317:bool)
        n373 = property on="med 1 PLC" class="Str"("Visible"=w345) -> ()  [unwired: 2 in, 2 out]
        n374 = property on="filt" class="Str"("Visible"=FALSE) -> ()  [unwired: 2 in, 2 out]
        n375 = property on="fast 0.1 PLC" class="Str"("Visible"=w343) -> ()  [unwired: 2 in, 2 out]
        n376 = Not Or(1:w320, 2:w326) -> (0:w325:bool)
        n377 = Select(t=FALSE, s=w325, f=w317) -> (s? t:f=w323:bool)
        n378 = property on="auto" class="Str"("Visible"=w323) -> ()  [unwired: 2 in, 2 out]
        n379 = property on="EX TRIG" class="Bool"("DisabledEnum"=w339) -> ()  [unwired: 2 in, 2 out]
        n380 = property on="TRIG" class="Bool"("DisabledEnum"=w339) -> ()  [unwired: 2 in, 2 out]
        n381 = property on="RECALL" class="Bool"("DisabledEnum"=w339) -> ()  [unwired: 2 in, 2 out]
        n382 = property on="RESTR" class="Bool"("DisabledEnum"=w339) -> ()  [unwired: 2 in, 2 out]
        n383 = Equal To 0?(x=w329) -> (x = 0?=w330:bool)
        n384 = property on="VALUE" class="Bool"("DisabledEnum"=w339) -> ()  [unwired: 2 in, 2 out]
        n385 = property on="RATE" class="Bool"("DisabledEnum"=w339) -> ()  [unwired: 2 in, 2 out]
        n386 = property on="AUTO" class="Bool"("DisabledEnum"=w339) -> ()  [unwired: 2 in, 2 out]
        n387 = property on="STORE" class="Bool"("DisabledEnum"=w339) -> ()  [unwired: 2 in, 2 out]
        n388 = property on="FILT" class="Bool"("DisabledEnum"=w339) -> ()  [unwired: 2 in, 2 out]
        n389 = property on="shift" class="Str"("Visible"=w341) -> ()  [unwired: 2 in, 2 out]
        n390 = case shown="True" w330 {
          tunnel: w327 -> [_ w356]
          tunnel: w321 -> [_ w355]
          tunnel: [w347 w354] -> w332
          tunnel: w329 -> [w346 _]
          frame False {
            n391 = Quotient & Remainder(x=w346, y=2) -> (x-y*floor(x/y)=w352:i32)  [unwired: 1 out]
            n392 = Equal?(x=w352, y=1 ("x")) -> (x = y?=w350:bool)
            n393 = Select(t="ON", s=w350, f="OFF") -> (s? t:f=w347:string)
          }
          frame True {
            n394 = case shown="3" w356 {
              tunnel: w355 -> [_ w362 w367 w372 w377]
              tunnel: ["Default" w358 w363 w368 w373] -> w354
              frame Default {
              }
              frame 0 {
                n395 = Unbundle By Name(w362) -> ("Analog1"=w359:bool)
                n396 = Select(t="ON", s=w359, f="OFF") -> (s? t:f=w358:string)
              }
              frame 2 {
                n397 = Unbundle By Name(w367) -> ("Analog2"=w364:bool)
                n398 = Select(t="ON", s=w364, f="OFF") -> (s? t:f=w363:string)
              }
              frame 3 {
                n399 = Unbundle By Name(w372) -> ("Analog temp 1"=w369:bool)
                n400 = Select(t="ON", s=w369, f="OFF") -> (s? t:f=w368:string)
              }
              frame 4 {
                n401 = Unbundle By Name(w377) -> ("Analog temp 1"=w375:bool, "Analog temp 2"=w374:bool, "Sens"=w376:bool)
                n402 = case shown="True" w376 {
                  tunnel: w375 -> [_ w383]
                  tunnel: w374 -> [w379 _]
                  tunnel: [w378 w382] -> w373
                  frame True {
                    n403 = Select(t="ON", s=w379, f="OFF") -> (s? t:f=w378:string)
                  }
                  frame False {
                    n404 = Select(t="ON", s=w383, f="OFF") -> (s? t:f=w382:string)
                  }
                }
              }
            }
          }
        }
        n405 = call "11-type_analog_bis.vi"("Count in"=w329, "this"=w336, "button"=w338, "Cluster"=w321) -> ("Count out"=w331:i32, "next state"=w335:i32, "Cluster 2"=w337:T7)
        n406 = case shown="3" w327 {
          tunnel: w321 -> [_ _ _ w390 w393]
          frame Default {
          }
          frame 0 {
            n407 = property on="CH1" class="Str"("Visible"=TRUE) -> ()  [unwired: 2 in, 2 out]
            n408 = property on="CH2" class="Str"("Visible"=FALSE) -> ()  [unwired: 2 in, 2 out]
          }
          frame 2 {
            n409 = property on="CH1" class="Str"("Visible"=FALSE) -> ()  [unwired: 2 in, 2 out]
            n410 = property on="CH2" class="Str"("Visible"=TRUE) -> ()  [unwired: 2 in, 2 out]
          }
          frame 3 {
            n411 = Unbundle By Name(w390) -> ("Sens"=w392:bool)
            n412 = property on="CH2" class="Str"("Visible"=FALSE) -> ()  [unwired: 2 in, 2 out]
            n413 = property on="CH1" class="Str"("Visible"=w392) -> ()  [unwired: 2 in, 2 out]
          }
          frame 4 {
            n414 = Unbundle By Name(w393) -> ("Sens"=w394:bool)
            n415 = property on="CH2" class="Str"("Visible"=w394) -> ()  [unwired: 2 in, 2 out]
            n416 = property on="CH1" class="Str"("Visible"=FALSE) -> ()  [unwired: 2 in, 2 out]
          }
        }
        n417 = Concatenate Strings("Stato undici " ("DISPLAY"), w332) -> (w334:string)
        n418 = property on="RIGHTARR" class="Bool"("DisabledEnum"=w340) -> ()  [unwired: 2 in, 2 out]
        n419 = property on="ENTER" class="Bool"("DisabledEnum"=w340) -> ()  [unwired: 2 in, 2 out]
        n420 = property on="RANGE UP" class="Bool"("DisabledEnum"=w340) -> ()  [unwired: 2 in, 2 out]
        n421 = property on="TEMP 2" class="Bool"("DisabledEnum"=w340) -> ()  [unwired: 2 in, 2 out]
        n422 = property on="TEMP1" class="Bool"("DisabledEnum"=w340) -> ()  [unwired: 2 in, 2 out]
        n423 = property on="LEFTARR" class="Bool"("DisabledEnum"=w340) -> ()  [unwired: 2 in, 2 out]
        n424 = property on="EXIT" class="Bool"("DisabledEnum"=w340) -> ()  [unwired: 2 in, 2 out]
        n425 = property on="DCV2" class="Bool"("DisabledEnum"=w340) -> ()  [unwired: 2 in, 2 out]
        n426 = property on="RANGE DOWN" class="Bool"("DisabledEnum"=w340) -> ()  [unwired: 2 in, 2 out]
        n427 = property on="DCV1" class="Bool"("DisabledEnum"=w340) -> ()  [unwired: 2 in, 2 out]
        n428 = local write "DISPLAY"(w334) -> ()
      }
      frame 12 {
        w411 = T3."Disabled and Grayed Out" ("Disabled")
        w412 = T3."Enabled" ("Disabled")
        n429 = property on="SCAN" class="Bool"("DisabledEnum"=w411) -> ()  [unwired: 2 in, 2 out]
        n430 = property on="ON/OFF" class="Bool"("DisabledEnum"=w411) -> ()  [unwired: 2 in, 2 out]
        n431 = property on="REL" class="Bool"("DisabledEnum"=w411) -> ()  [unwired: 2 in, 2 out]
        n432 = property on="DIGITS" class="Bool"("DisabledEnum"=w411) -> ()  [unwired: 2 in, 2 out]
        n433 = property on="SAVE" class="Bool"("DisabledEnum"=w411) -> ()  [unwired: 2 in, 2 out]
        n434 = property on="ACAL" class="Bool"("DisabledEnum"=w411) -> ()  [unwired: 2 in, 2 out]
        n435 = property on="SHIFT" class="Bool"("DisabledEnum"=w411) -> ()  [unwired: 2 in, 2 out]
        n436 = property on="V1/V2" class="Bool"("DisabledEnum"=w411) -> ()  [unwired: 2 in, 2 out]
        n437 = property on="STEP" class="Bool"("DisabledEnum"=w411) -> ()  [unwired: 2 in, 2 out]
        n438 = Unbundle By Name(w400) -> ("prevState"=w399:i32, "Rate"=w421:u16)
        n439 = Equal To 0?(x=w421) -> (x = 0?=w419:bool)
        n440 = Equal?(x=u16 1, y=w421) -> (x = y?=w418:bool)
        n441 = Equal?(x=w421, y=u16 2) -> (x = y?=w420:bool)
        n442 = property on="EX TRIG" class="Bool"("DisabledEnum"=w411) -> ()  [unwired: 2 in, 2 out]
        n443 = property on="TRIG" class="Bool"("DisabledEnum"=w411) -> ()  [unwired: 2 in, 2 out]
        n444 = property on="RECALL" class="Bool"("DisabledEnum"=w411) -> ()  [unwired: 2 in, 2 out]
        n445 = property on="RESTR" class="Bool"("DisabledEnum"=w411) -> ()  [unwired: 2 in, 2 out]
        n446 = property on="VALUE" class="Bool"("DisabledEnum"=w411) -> ()  [unwired: 2 in, 2 out]
        n447 = property on="RATE" class="Bool"("DisabledEnum"=w411) -> ()  [unwired: 2 in, 2 out]
        n448 = property on="AUTO" class="Bool"("DisabledEnum"=w411) -> ()  [unwired: 2 in, 2 out]
        n449 = property on="STORE" class="Bool"("DisabledEnum"=w411) -> ()  [unwired: 2 in, 2 out]
        n450 = property on="FILT" class="Bool"("DisabledEnum"=w411) -> ()  [unwired: 2 in, 2 out]
        n451 = property on="shift" class="Str"("Visible"=w413) -> ()  [unwired: 2 in, 2 out]
        n452 = property on="slow 5 PLC" class="Str"("Visible"=w419) -> ()  [unwired: 2 in, 2 out]
        n453 = property on="med 1 PLC" class="Str"("Visible"=w420) -> ()  [unwired: 2 in, 2 out]
        n454 = property on="fast 0.1 PLC" class="Str"("Visible"=w418) -> ()  [unwired: 2 in, 2 out]
        n455 = property on="filt" class="Str"("Visible"=FALSE) -> ()  [unwired: 2 in, 2 out]
        n456 = Unbundle By Name(w400) -> ("Auto2"=w403:bool, "Auto1"=w402:bool)
        n457 = call "12-type_digital.vi"("this"=w415, "button"=w416, "settings in"=w400) -> ("next state"=w414:i32, "settings in"=w410:T7)
        n458 = Equal To 0?(x=w399) -> (x = 0?=w407:bool)
        n459 = Equal?(x=w399, y=2) -> (x = y?=w404:bool)
        n460 = case shown="4" w399 {
          tunnel: w400 -> [_ _ _ w427 w430]
          frame Default {
          }
          frame 0 {
            n461 = property on="CH1" class="Str"("Visible"=TRUE) -> ()  [unwired: 2 in, 2 out]
            n462 = property on="CH2" class="Str"("Visible"=FALSE) -> ()  [unwired: 2 in, 2 out]
          }
          frame 2 {
            n463 = property on="CH1" class="Str"("Visible"=FALSE) -> ()  [unwired: 2 in, 2 out]
            n464 = property on="CH2" class="Str"("Visible"=TRUE) -> ()  [unwired: 2 in, 2 out]
          }
          frame 3 {
            n465 = Unbundle By Name(w427) -> ("Sens"=w429:bool)
            n466 = property on="CH2" class="Str"("Visible"=FALSE) -> ()  [unwired: 2 in, 2 out]
            n467 = property on="CH1" class="Str"("Visible"=w429) -> ()  [unwired: 2 in, 2 out]
          }
          frame 4 {
            n468 = Unbundle By Name(w430) -> ("Sens"=w431:bool)
            n469 = property on="CH2" class="Str"("Visible"=w431) -> ()  [unwired: 2 in, 2 out]
            n470 = property on="CH1" class="Str"("Visible"=FALSE) -> ()  [unwired: 2 in, 2 out]
          }
        }
        n471 = Select(t=w403, s=w404, f=w402) -> (s? t:f=w401:bool)
        n472 = Not Or(1:w404, 2:w407) -> (0:w406:bool)
        n473 = Select(t=FALSE, s=w406, f=w401) -> (s? t:f=w398:bool)
        n474 = property on="auto" class="Str"("Visible"=w398) -> ()  [unwired: 2 in, 2 out]
        n475 = property on="RIGHTARR" class="Bool"("DisabledEnum"=w412) -> ()  [unwired: 2 in, 2 out]
        n476 = property on="ENTER" class="Bool"("DisabledEnum"=w412) -> ()  [unwired: 2 in, 2 out]
        n477 = property on="RANGE UP" class="Bool"("DisabledEnum"=w412) -> ()  [unwired: 2 in, 2 out]
        n478 = property on="TEMP 2" class="Bool"("DisabledEnum"=w412) -> ()  [unwired: 2 in, 2 out]
        n479 = property on="TEMP1" class="Bool"("DisabledEnum"=w412) -> ()  [unwired: 2 in, 2 out]
        n480 = property on="LEFTARR" class="Bool"("DisabledEnum"=w412) -> ()  [unwired: 2 in, 2 out]
        n481 = property on="EXIT" class="Bool"("DisabledEnum"=w412) -> ()  [unwired: 2 in, 2 out]
        n482 = property on="DCV2" class="Bool"("DisabledEnum"=w412) -> ()  [unwired: 2 in, 2 out]
        n483 = property on="RANGE DOWN" class="Bool"("DisabledEnum"=w412) -> ()  [unwired: 2 in, 2 out]
        n484 = property on="DCV1" class="Bool"("DisabledEnum"=w412) -> ()  [unwired: 2 in, 2 out]
        n485 = local write "DISPLAY"("Stato dodici" ("Label.Text")) -> ()
      }
      frame 13 {
        w458 = T3."Disabled and Grayed Out" ("Disabled")
        w459 = T3."Enabled" ("Disabled")
        n486 = Unbundle By Name(w436) -> ("prevState"=w438:i32, "Rate"=w437:u16)
        n487 = Unbundle By Name(w436) -> ("Auto2"=w441:bool, "Auto1"=w440:bool)
        n488 = property on="SCAN" class="Bool"("DisabledEnum"=w458) -> ()  [unwired: 2 in, 2 out]
        n489 = property on="ON/OFF" class="Bool"("DisabledEnum"=w458) -> ()  [unwired: 2 in, 2 out]
        n490 = property on="REL" class="Bool"("DisabledEnum"=w458) -> ()  [unwired: 2 in, 2 out]
        n491 = property on="DIGITS" class="Bool"("DisabledEnum"=w458) -> ()  [unwired: 2 in, 2 out]
        n492 = property on="SAVE" class="Bool"("DisabledEnum"=w458) -> ()  [unwired: 2 in, 2 out]
        n493 = property on="ACAL" class="Bool"("DisabledEnum"=w458) -> ()  [unwired: 2 in, 2 out]
        n494 = property on="SHIFT" class="Bool"("DisabledEnum"=w458) -> ()  [unwired: 2 in, 2 out]
        n495 = property on="V1/V2" class="Bool"("DisabledEnum"=w458) -> ()  [unwired: 2 in, 2 out]
        n496 = property on="STEP" class="Bool"("DisabledEnum"=w458) -> ()  [unwired: 2 in, 2 out]
        n497 = Equal To 0?(x=w437) -> (x = 0?=w463:bool)
        n498 = Equal?(x=u16 1, y=w437) -> (x = y?=w462:bool)
        n499 = Equal?(x=w437, y=u16 2) -> (x = y?=w464:bool)
        n500 = Equal To 0?(x=w438) -> (x = 0?=w445:bool)
        n501 = Equal?(x=w438, y=2) -> (x = y?=w442:bool)
        n502 = Select(t=w441, s=w442, f=w440) -> (s? t:f=w439:bool)
        n503 = property on="slow 5 PLC" class="Str"("Visible"=w463) -> ()  [unwired: 2 in, 2 out]
        n504 = property on="med 1 PLC" class="Str"("Visible"=w464) -> ()  [unwired: 2 in, 2 out]
        n505 = Not Or(1:w442, 2:w445) -> (0:w444:bool)
        n506 = property on="filt" class="Str"("Visible"=FALSE) -> ()  [unwired: 2 in, 2 out]
        n507 = property on="fast 0.1 PLC" class="Str"("Visible"=w462) -> ()  [unwired: 2 in, 2 out]
        n508 = Select(t=FALSE, s=w444, f=w439) -> (s? t:f=w435:bool)
        n509 = property on="auto" class="Str"("Visible"=w435) -> ()  [unwired: 2 in, 2 out]
        n510 = Unbundle By Name(w436) -> ("prevState"=w453:i32)
        n511 = property on="EX TRIG" class="Bool"("DisabledEnum"=w458) -> ()  [unwired: 2 in, 2 out]
        n512 = property on="TRIG" class="Bool"("DisabledEnum"=w458) -> ()  [unwired: 2 in, 2 out]
        n513 = property on="RECALL" class="Bool"("DisabledEnum"=w458) -> ()  [unwired: 2 in, 2 out]
        n514 = property on="RESTR" class="Bool"("DisabledEnum"=w458) -> ()  [unwired: 2 in, 2 out]
        n515 = Equal To 0?(x=w447) -> (x = 0?=w448:bool)
        n516 = property on="VALUE" class="Bool"("DisabledEnum"=w458) -> ()  [unwired: 2 in, 2 out]
        n517 = property on="RATE" class="Bool"("DisabledEnum"=w458) -> ()  [unwired: 2 in, 2 out]
        n518 = property on="AUTO" class="Bool"("DisabledEnum"=w458) -> ()  [unwired: 2 in, 2 out]
        n519 = property on="STORE" class="Bool"("DisabledEnum"=w458) -> ()  [unwired: 2 in, 2 out]
        n520 = property on="FILT" class="Bool"("DisabledEnum"=w458) -> ()  [unwired: 2 in, 2 out]
        n521 = property on="shift" class="Str"("Visible"=w460) -> ()  [unwired: 2 in, 2 out]
        n522 = case shown="True" w448 {
          tunnel: w453 -> [_ w475]
          tunnel: w436 -> [_ w474]
          tunnel: [w466 w473] -> w450
          tunnel: w447 -> [w465 _]
          frame False {
            n523 = Quotient & Remainder(x=w465, y=2) -> (x-y*floor(x/y)=w471:i32)  [unwired: 1 out]
            n524 = Equal?(x=w471, y=1 ("x")) -> (x = y?=w469:bool)
            n525 = Select(t="ON", s=w469, f="OFF") -> (s? t:f=w466:string)
          }
          frame True {
            n526 = case shown="2" w475 {
              tunnel: w474 -> [_ w481 w486 w491 w496]
              tunnel: ["Default" w477 w482 w487 w492] -> w473
              frame Default {
              }
              frame 0 {
                n527 = Unbundle By Name(w481) -> ("Digital1"=w478:bool)
                n528 = Select(t="ON", s=w478, f="OFF") -> (s? t:f=w477:string)
              }
              frame 2 {
                n529 = Unbundle By Name(w486) -> ("Digital2"=w483:bool)
                n530 = Select(t="ON", s=w483, f="OFF") -> (s? t:f=w482:string)
              }
              frame 3 {
                n531 = Unbundle By Name(w491) -> ("Digital temp 1"=w488:bool)
                n532 = Select(t="ON", s=w488, f="OFF") -> (s? t:f=w487:string)
              }
              frame 4 {
                n533 = Unbundle By Name(w496) -> ("Digital temp 1"=w494:bool, "Digital temp 2"=w493:bool, "Sens"=w495:bool)
                n534 = case shown="True" w495 {
                  tunnel: w494 -> [_ w502]
                  tunnel: w493 -> [w498 _]
                  tunnel: [w497 w501] -> w492
                  frame True {
                    n535 = Select(t="ON", s=w498, f="OFF") -> (s? t:f=w497:string)
                  }
                  frame False {
                    n536 = Select(t="ON", s=w502, f="OFF") -> (s? t:f=w501:string)
                  }
                }
              }
            }
          }
        }
        n537 = call "13-type_digital_bis.vi"("this"=w455, "Count in"=w447, "button"=w457, "Cluster"=w436) -> ("next state"=w454:i32, "Count out"=w449:i32, "Cluster 2"=w456:T7)
        n538 = case shown="3" w438 {
          tunnel: w436 -> [_ _ _ w509 w512]
          frame Default {
          }
          frame 0 {
            n539 = property on="CH1" class="Str"("Visible"=TRUE) -> ()  [unwired: 2 in, 2 out]
            n540 = property on="CH2" class="Str"("Visible"=FALSE) -> ()  [unwired: 2 in, 2 out]
          }
          frame 2 {
            n541 = property on="CH1" class="Str"("Visible"=FALSE) -> ()  [unwired: 2 in, 2 out]
            n542 = property on="CH2" class="Str"("Visible"=TRUE) -> ()  [unwired: 2 in, 2 out]
          }
          frame 3 {
            n543 = Unbundle By Name(w509) -> ("Sens"=w511:bool)
            n544 = property on="CH2" class="Str"("Visible"=FALSE) -> ()  [unwired: 2 in, 2 out]
            n545 = property on="CH1" class="Str"("Visible"=w511) -> ()  [unwired: 2 in, 2 out]
          }
          frame 4 {
            n546 = Unbundle By Name(w512) -> ("Sens"=w513:bool)
            n547 = property on="CH2" class="Str"("Visible"=w513) -> ()  [unwired: 2 in, 2 out]
            n548 = property on="CH1" class="Str"("Visible"=FALSE) -> ()  [unwired: 2 in, 2 out]
          }
        }
        n549 = Concatenate Strings("Stato tredici " ("DISPLAY"), w450) -> (w452:string)
        n550 = property on="RIGHTARR" class="Bool"("DisabledEnum"=w459) -> ()  [unwired: 2 in, 2 out]
        n551 = property on="ENTER" class="Bool"("DisabledEnum"=w459) -> ()  [unwired: 2 in, 2 out]
        n552 = property on="RANGE UP" class="Bool"("DisabledEnum"=w459) -> ()  [unwired: 2 in, 2 out]
        n553 = property on="TEMP 2" class="Bool"("DisabledEnum"=w459) -> ()  [unwired: 2 in, 2 out]
        n554 = property on="TEMP1" class="Bool"("DisabledEnum"=w459) -> ()  [unwired: 2 in, 2 out]
        n555 = property on="LEFTARR" class="Bool"("DisabledEnum"=w459) -> ()  [unwired: 2 in, 2 out]
        n556 = property on="EXIT" class="Bool"("DisabledEnum"=w459) -> ()  [unwired: 2 in, 2 out]
        n557 = property on="DCV2" class="Bool"("DisabledEnum"=w459) -> ()  [unwired: 2 in, 2 out]
        n558 = property on="RANGE DOWN" class="Bool"("DisabledEnum"=w459) -> ()  [unwired: 2 in, 2 out]
        n559 = property on="DCV1" class="Bool"("DisabledEnum"=w459) -> ()  [unwired: 2 in, 2 out]
        n560 = local write "DISPLAY"(w452) -> ()
      }
      frame 14 {
        w516 = T3."Disabled and Grayed Out" ("Disabled")
        w542 = T3."Enabled" ("Disabled")
        n561 = Unbundle By Name(w520) -> ("prevState"=w522:i32, "Rate"=w521:u16)
        n562 = Unbundle By Name(w520) -> ("Auto2"=w525:bool, "Auto1"=w524:bool)
        n563 = property on="SCAN" class="Bool"("DisabledEnum"=w516) -> ()  [unwired: 2 in, 2 out]
        n564 = property on="ON/OFF" class="Bool"("DisabledEnum"=w516) -> ()  [unwired: 2 in, 2 out]
        n565 = property on="REL" class="Bool"("DisabledEnum"=w516) -> ()  [unwired: 2 in, 2 out]
        n566 = property on="DIGITS" class="Bool"("DisabledEnum"=w516) -> ()  [unwired: 2 in, 2 out]
        n567 = property on="SAVE" class="Bool"("DisabledEnum"=w516) -> ()  [unwired: 2 in, 2 out]
        n568 = property on="ACAL" class="Bool"("DisabledEnum"=w516) -> ()  [unwired: 2 in, 2 out]
        n569 = property on="SHIFT" class="Bool"("DisabledEnum"=w516) -> ()  [unwired: 2 in, 2 out]
        n570 = property on="V1/V2" class="Bool"("DisabledEnum"=w516) -> ()  [unwired: 2 in, 2 out]
        n571 = property on="STEP" class="Bool"("DisabledEnum"=w516) -> ()  [unwired: 2 in, 2 out]
        n572 = Equal To 0?(x=w521) -> (x = 0?=w546:bool)
        n573 = Equal?(x=u16 1, y=w521) -> (x = y?=w545:bool)
        n574 = Equal?(x=w521, y=u16 2) -> (x = y?=w547:bool)
        n575 = Equal To 0?(x=w522) -> (x = 0?=w529:bool)
        n576 = Equal?(x=w522, y=2) -> (x = y?=w526:bool)
        n577 = Select(t=w525, s=w526, f=w524) -> (s? t:f=w523:bool)
        n578 = property on="LEFTARR" class="Bool"("DisabledEnum"=w516) -> ()  [unwired: 2 in, 2 out]
        n579 = property on="slow 5 PLC" class="Str"("Visible"=w546) -> ()  [unwired: 2 in, 2 out]
        n580 = property on="med 1 PLC" class="Str"("Visible"=w547) -> ()  [unwired: 2 in, 2 out]
        n581 = Not Or(1:w526, 2:w529) -> (0:w528:bool)
        n582 = property on="filt" class="Str"("Visible"=FALSE) -> ()  [unwired: 2 in, 2 out]
        n583 = property on="fast 0.1 PLC" class="Str"("Visible"=w545) -> ()  [unwired: 2 in, 2 out]
        n584 = Select(t=FALSE, s=w528, f=w523) -> (s? t:f=w519:bool)
        n585 = property on="RIGHTARR" class="Bool"("DisabledEnum"=w516) -> ()  [unwired: 2 in, 2 out]
        n586 = property on="auto" class="Str"("Visible"=w519) -> ()  [unwired: 2 in, 2 out]
        n587 = Unbundle By Name(w520) -> ("prevState"=w537:i32)
        n588 = property on="EX TRIG" class="Bool"("DisabledEnum"=w516) -> ()  [unwired: 2 in, 2 out]
        n589 = property on="TRIG" class="Bool"("DisabledEnum"=w516) -> ()  [unwired: 2 in, 2 out]
        n590 = property on="RECALL" class="Bool"("DisabledEnum"=w516) -> ()  [unwired: 2 in, 2 out]
        n591 = property on="RESTR" class="Bool"("DisabledEnum"=w516) -> ()  [unwired: 2 in, 2 out]
        n592 = Equal?(x=-1, y=w531) -> (x = y?=w532:bool)
        n593 = property on="VALUE" class="Bool"("DisabledEnum"=w516) -> ()  [unwired: 2 in, 2 out]
        n594 = property on="RATE" class="Bool"("DisabledEnum"=w516) -> ()  [unwired: 2 in, 2 out]
        n595 = property on="AUTO" class="Bool"("DisabledEnum"=w516) -> ()  [unwired: 2 in, 2 out]
        n596 = property on="STORE" class="Bool"("DisabledEnum"=w516) -> ()  [unwired: 2 in, 2 out]
        n597 = property on="FILT" class="Bool"("DisabledEnum"=w516) -> ()  [unwired: 2 in, 2 out]
        n598 = property on="shift" class="Str"("Visible"=w543) -> ()  [unwired: 2 in, 2 out]
        n599 = case shown="True" w532 {
          tunnel: w537 -> [_ w552]
          tunnel: w520 -> [_ w551]
          tunnel: [w548 w550] -> w534
          tunnel: w531 -> [w549 _]
          frame False {
            n600 = Number To Decimal String(number=w549) -> (decimal integer string=w548:string)  [unwired: 1 in]
          }
          frame True {
            n601 = case shown="4" w552 {
              tunnel: w551 -> [_ w556 w559 w562 w567]
              tunnel: ["Default" w554 w557 w560 w563] -> w550
              frame Default {
              }
              frame 0 {
                n602 = Unbundle By Name(w556) -> ("Window1"=w555:u16)
                n603 = Number To Decimal String(number=w555) -> (decimal integer string=w554:string)  [unwired: 1 in]
              }
              frame 2 {
                n604 = Unbundle By Name(w559) -> ("Window2"=w558:enum16{"0,01%", "0,1%", "1%", "10%", "None"})
                n605 = Number To Decimal String(number=w558) -> (decimal integer string=w557:string)  [unwired: 1 in]
              }
              frame 3 {
                n606 = Unbundle By Name(w562) -> ("Window temp 1"=w561:enum16{"0,01%", "0,1%", "1%", "10%", "None"})
                n607 = Number To Decimal String(number=w561) -> (decimal integer string=w560:string)  [unwired: 1 in]
              }
              frame 4 {
                n608 = Unbundle By Name(w567) -> ("Window temp 1"=w565:enum16{"0,01%", "0,1%", "1%", "10%", "None"}, "Window temp 2"=w564:enum16{"0,01%", "0,1%", "1%", "10%", "None"}, "Sens"=w566:bool)
                n609 = case shown="False" w566 {
                  tunnel: w565 -> [_ w573]
                  tunnel: w564 -> [w569 _]
                  tunnel: [w568 w570] -> w563
                  frame True {
                    n610 = Number To Decimal String(number=w569) -> (decimal integer string=w568:string)  [unwired: 1 in]
                  }
                  frame False {
                    w572 = enum16{"0,01%", "0,1%", "1%", "10%", "None"}."None"  # Window1
                    n611 = property on="number as enum" class="Enum (strict)"() -> ("RingText.Text"=w570:string)  [unwired: 2 in, 2 out]
                    n612 = call "Number To Enum.vim"("number"=w573, "enum type"=w572) -> ("number as enum"=→"number as enum":enum16{"0,01%", "0,1%", "1%", "10%", "None"})
                  }
                }
              }
            }
          }
        }
        n613 = call "14-type_window.vi"("this"=w539, "window in"=w531, "button"=w541, "Cluster"=w520) -> ("next state"=w538:i32, "window out"=w533:i32, "Cluster 2"=w540:T8)
        n614 = case shown="4" w522 {
          tunnel: w520 -> [_ _ _ w578 w581]
          frame Default {
          }
          frame 0 {
            n615 = property on="CH1" class="Str"("Visible"=TRUE) -> ()  [unwired: 2 in, 2 out]
            n616 = property on="CH2" class="Str"("Visible"=FALSE) -> ()  [unwired: 2 in, 2 out]
          }
          frame 2 {
            n617 = property on="CH1" class="Str"("Visible"=FALSE) -> ()  [unwired: 2 in, 2 out]
            n618 = property on="CH2" class="Str"("Visible"=TRUE) -> ()  [unwired: 2 in, 2 out]
          }
          frame 3 {
            n619 = Unbundle By Name(w578) -> ("Sens"=w580:bool)
            n620 = property on="CH2" class="Str"("Visible"=FALSE) -> ()  [unwired: 2 in, 2 out]
            n621 = property on="CH1" class="Str"("Visible"=w580) -> ()  [unwired: 2 in, 2 out]
          }
          frame 4 {
            n622 = Unbundle By Name(w581) -> ("Sens"=w582:bool)
            n623 = property on="CH2" class="Str"("Visible"=w582) -> ()  [unwired: 2 in, 2 out]
            n624 = property on="CH1" class="Str"("Visible"=FALSE) -> ()  [unwired: 2 in, 2 out]
          }
        }
        n625 = property on="ENTER" class="Bool"("DisabledEnum"=w542) -> ()  [unwired: 2 in, 2 out]
        n626 = Concatenate Strings("Stato quattordici " ("DISPLAY"), w534) -> (w536:string)
        n627 = property on="TEMP 2" class="Bool"("DisabledEnum"=w542) -> ()  [unwired: 2 in, 2 out]
        n628 = property on="TEMP1" class="Bool"("DisabledEnum"=w542) -> ()  [unwired: 2 in, 2 out]
        n629 = property on="RANGE UP" class="Bool"("DisabledEnum"=w542) -> ()  [unwired: 2 in, 2 out]
        n630 = property on="EXIT" class="Bool"("DisabledEnum"=w542) -> ()  [unwired: 2 in, 2 out]
        n631 = property on="DCV2" class="Bool"("DisabledEnum"=w542) -> ()  [unwired: 2 in, 2 out]
        n632 = property on="DCV1" class="Bool"("DisabledEnum"=w542) -> ()  [unwired: 2 in, 2 out]
        n633 = property on="RANGE DOWN" class="Bool"("DisabledEnum"=w542) -> ()  [unwired: 2 in, 2 out]
        n634 = local write "DISPLAY"(w536) -> ()
      }
      frame 15 {
        w595 = T3."Disabled and Grayed Out" ("Disabled")
        w596 = T3."Enabled" ("Disabled")
        n635 = Unbundle By Name(w588) -> ("prevState"=w590:i32, "Rate"=w589:u16)
        n636 = property on="SCAN" class="Bool"("DisabledEnum"=w595) -> ()  [unwired: 2 in, 2 out]
        n637 = property on="ON/OFF" class="Bool"("DisabledEnum"=w595) -> ()  [unwired: 2 in, 2 out]
        n638 = property on="REL" class="Bool"("DisabledEnum"=w595) -> ()  [unwired: 2 in, 2 out]
        n639 = property on="DIGITS" class="Bool"("DisabledEnum"=w595) -> ()  [unwired: 2 in, 2 out]
        n640 = property on="SAVE" class="Bool"("DisabledEnum"=w595) -> ()  [unwired: 2 in, 2 out]
        n641 = property on="ACAL" class="Bool"("DisabledEnum"=w595) -> ()  [unwired: 2 in, 2 out]
        n642 = property on="SHIFT" class="Bool"("DisabledEnum"=w595) -> ()  [unwired: 2 in, 2 out]
        n643 = property on="V1/V2" class="Bool"("DisabledEnum"=w595) -> ()  [unwired: 2 in, 2 out]
        n644 = property on="STEP" class="Bool"("DisabledEnum"=w595) -> ()  [unwired: 2 in, 2 out]
        n645 = Equal To 0?(x=w589) -> (x = 0?=w600:bool)
        n646 = Equal?(x=u16 1, y=w589) -> (x = y?=w599:bool)
        n647 = Equal?(x=w589, y=u16 2) -> (x = y?=w601:bool)
        n648 = property on="slow 5 PLC" class="Str"("Visible"=w600) -> ()  [unwired: 2 in, 2 out]
        n649 = property on="med 1 PLC" class="Str"("Visible"=w601) -> ()  [unwired: 2 in, 2 out]
        n650 = property on="filt" class="Str"("Visible"=FALSE) -> ()  [unwired: 2 in, 2 out]
        n651 = property on="fast 0.1 PLC" class="Str"("Visible"=w599) -> ()  [unwired: 2 in, 2 out]
        n652 = property on="EX TRIG" class="Bool"("DisabledEnum"=w595) -> ()  [unwired: 2 in, 2 out]
        n653 = property on="TRIG" class="Bool"("DisabledEnum"=w595) -> ()  [unwired: 2 in, 2 out]
        n654 = property on="RECALL" class="Bool"("DisabledEnum"=w595) -> ()  [unwired: 2 in, 2 out]
        n655 = property on="RESTR" class="Bool"("DisabledEnum"=w595) -> ()  [unwired: 2 in, 2 out]
        n656 = property on="VALUE" class="Bool"("DisabledEnum"=w595) -> ()  [unwired: 2 in, 2 out]
        n657 = property on="RATE" class="Bool"("DisabledEnum"=w595) -> ()  [unwired: 2 in, 2 out]
        n658 = property on="AUTO" class="Bool"("DisabledEnum"=w595) -> ()  [unwired: 2 in, 2 out]
        n659 = property on="STORE" class="Bool"("DisabledEnum"=w595) -> ()  [unwired: 2 in, 2 out]
        n660 = property on="FILT" class="Bool"("DisabledEnum"=w595) -> ()  [unwired: 2 in, 2 out]
        n661 = property on="shift" class="Str"("Visible"=w597) -> ()  [unwired: 2 in, 2 out]
        n662 = call "15-tcoupl_units.vi"("this"=w592, "button"=w594, "Cluster"=w588) -> ("next state"=w591:i32, "Cluster 2"=w593:T1)
        n663 = case shown="3" w590 {
          tunnel: w588 -> [_ _ _ w606 w609]
          frame Default {
          }
          frame 0 {
            n664 = property on="CH1" class="Str"("Visible"=TRUE) -> ()  [unwired: 2 in, 2 out]
            n665 = property on="CH2" class="Str"("Visible"=FALSE) -> ()  [unwired: 2 in, 2 out]
          }
          frame 2 {
            n666 = property on="CH1" class="Str"("Visible"=FALSE) -> ()  [unwired: 2 in, 2 out]
            n667 = property on="CH2" class="Str"("Visible"=TRUE) -> ()  [unwired: 2 in, 2 out]
          }
          frame 3 {
            n668 = Unbundle By Name(w606) -> ("Sens"=w608:bool)
            n669 = property on="CH2" class="Str"("Visible"=FALSE) -> ()  [unwired: 2 in, 2 out]
            n670 = property on="CH1" class="Str"("Visible"=w608) -> ()  [unwired: 2 in, 2 out]
          }
          frame 4 {
            n671 = Unbundle By Name(w609) -> ("Sens"=w610:bool)
            n672 = property on="CH2" class="Str"("Visible"=w610) -> ()  [unwired: 2 in, 2 out]
            n673 = property on="CH1" class="Str"("Visible"=FALSE) -> ()  [unwired: 2 in, 2 out]
          }
        }
        n674 = property on="RIGHTARR" class="Bool"("DisabledEnum"=w596) -> ()  [unwired: 2 in, 2 out]
        n675 = property on="ENTER" class="Bool"("DisabledEnum"=w596) -> ()  [unwired: 2 in, 2 out]
        n676 = property on="RANGE UP" class="Bool"("DisabledEnum"=w596) -> ()  [unwired: 2 in, 2 out]
        n677 = property on="TEMP 2" class="Bool"("DisabledEnum"=w596) -> ()  [unwired: 2 in, 2 out]
        n678 = property on="TEMP1" class="Bool"("DisabledEnum"=w596) -> ()  [unwired: 2 in, 2 out]
        n679 = property on="LEFTARR" class="Bool"("DisabledEnum"=w596) -> ()  [unwired: 2 in, 2 out]
        n680 = property on="EXIT" class="Bool"("DisabledEnum"=w596) -> ()  [unwired: 2 in, 2 out]
        n681 = property on="DCV2" class="Bool"("DisabledEnum"=w596) -> ()  [unwired: 2 in, 2 out]
        n682 = property on="RANGE DOWN" class="Bool"("DisabledEnum"=w596) -> ()  [unwired: 2 in, 2 out]
        n683 = property on="DCV1" class="Bool"("DisabledEnum"=w596) -> ()  [unwired: 2 in, 2 out]
        n684 = local write "DISPLAY"("Stato quindici " ("DISPLAY")) -> ()
      }
      frame 16 {
        w614 = T3."Disabled and Grayed Out" ("Disabled")
        w612 = T3."Enabled" ("Disabled")
        n685 = Unbundle By Name(w617) -> ("prevState"=w619:i32, "Rate"=w618:u16)
        n686 = property on="SCAN" class="Bool"("DisabledEnum"=w614) -> ()  [unwired: 2 in, 2 out]
        n687 = property on="ON/OFF" class="Bool"("DisabledEnum"=w614) -> ()  [unwired: 2 in, 2 out]
        n688 = property on="REL" class="Bool"("DisabledEnum"=w614) -> ()  [unwired: 2 in, 2 out]
        n689 = property on="DIGITS" class="Bool"("DisabledEnum"=w614) -> ()  [unwired: 2 in, 2 out]
        n690 = property on="SAVE" class="Bool"("DisabledEnum"=w614) -> ()  [unwired: 2 in, 2 out]
        n691 = property on="ACAL" class="Bool"("DisabledEnum"=w614) -> ()  [unwired: 2 in, 2 out]
        n692 = property on="SHIFT" class="Bool"("DisabledEnum"=w614) -> ()  [unwired: 2 in, 2 out]
        n693 = property on="V1/V2" class="Bool"("DisabledEnum"=w614) -> ()  [unwired: 2 in, 2 out]
        n694 = property on="STEP" class="Bool"("DisabledEnum"=w614) -> ()  [unwired: 2 in, 2 out]
        n695 = Equal To 0?(x=w618) -> (x = 0?=w633:bool)
        n696 = Equal?(x=u16 1, y=w618) -> (x = y?=w632:bool)
        n697 = Equal?(x=w618, y=u16 2) -> (x = y?=w634:bool)
        n698 = property on="slow 5 PLC" class="Str"("Visible"=w633) -> ()  [unwired: 2 in, 2 out]
        n699 = property on="med 1 PLC" class="Str"("Visible"=w634) -> ()  [unwired: 2 in, 2 out]
        n700 = property on="filt" class="Str"("Visible"=FALSE) -> ()  [unwired: 2 in, 2 out]
        n701 = property on="fast 0.1 PLC" class="Str"("Visible"=w632) -> ()  [unwired: 2 in, 2 out]
        n702 = property on="EX TRIG" class="Bool"("DisabledEnum"=w614) -> ()  [unwired: 2 in, 2 out]
        n703 = property on="TRIG" class="Bool"("DisabledEnum"=w614) -> ()  [unwired: 2 in, 2 out]
        n704 = property on="RECALL" class="Bool"("DisabledEnum"=w614) -> ()  [unwired: 2 in, 2 out]
        n705 = property on="RESTR" class="Bool"("DisabledEnum"=w614) -> ()  [unwired: 2 in, 2 out]
        n706 = Equal?(x=-1, y=w620) -> (x = y?=w621:bool)
        n707 = property on="VALUE" class="Bool"("DisabledEnum"=w614) -> ()  [unwired: 2 in, 2 out]
        n708 = property on="RATE" class="Bool"("DisabledEnum"=w614) -> ()  [unwired: 2 in, 2 out]
        n709 = property on="AUTO" class="Bool"("DisabledEnum"=w614) -> ()  [unwired: 2 in, 2 out]
        n710 = property on="STORE" class="Bool"("DisabledEnum"=w614) -> ()  [unwired: 2 in, 2 out]
        n711 = property on="FILT" class="Bool"("DisabledEnum"=w614) -> ()  [unwired: 2 in, 2 out]
        n712 = property on="shift" class="Str"("Visible"=w630) -> ()  [unwired: 2 in, 2 out]
        n713 = case shown="False" w621 {
          tunnel: w617 -> [_ w639]
          tunnel: [w635 w638] -> w623
          tunnel: w620 -> [w636 _]
          frame False {
            n714 = Number To Decimal String(number=w636) -> (decimal integer string=w635:string)  [unwired: 1 in]
          }
          frame True {
            n715 = Unbundle By Name(w639) -> ("Unit"=w637:enum16{"C", "K", "F"})
            n716 = Number To Decimal String(number=w637) -> (decimal integer string=w638:string)  [unwired: 1 in]
          }
        }
        n717 = call "16-tcoupl_units_bis.vi"("this"=w627, "unit in"=w620, "button"=w629, "Cluster"=w617) -> ("next state"=w626:i32, "unit out"=w622:i32, "Cluster 2"=w628:T1)
        n718 = case shown="0" w619 {
          tunnel: w617 -> [_ _ _ w644 w647]
          frame Default {
          }
          frame 0 {
            n719 = property on="CH1" class="Str"("Visible"=TRUE) -> ()  [unwired: 2 in, 2 out]
            n720 = property on="CH2" class="Str"("Visible"=FALSE) -> ()  [unwired: 2 in, 2 out]
          }
          frame 2 {
            n721 = property on="CH1" class="Str"("Visible"=FALSE) -> ()  [unwired: 2 in, 2 out]
            n722 = property on="CH2" class="Str"("Visible"=TRUE) -> ()  [unwired: 2 in, 2 out]
          }
          frame 3 {
            n723 = Unbundle By Name(w644) -> ("Sens"=w646:bool)
            n724 = property on="CH2" class="Str"("Visible"=FALSE) -> ()  [unwired: 2 in, 2 out]
            n725 = property on="CH1" class="Str"("Visible"=w646) -> ()  [unwired: 2 in, 2 out]
          }
          frame 4 {
            n726 = Unbundle By Name(w647) -> ("Sens"=w648:bool)
            n727 = property on="CH2" class="Str"("Visible"=w648) -> ()  [unwired: 2 in, 2 out]
            n728 = property on="CH1" class="Str"("Visible"=FALSE) -> ()  [unwired: 2 in, 2 out]
          }
        }
        n729 = property on="ENTER" class="Bool"("DisabledEnum"=w612) -> ()  [unwired: 2 in, 2 out]
        n730 = Concatenate Strings("Stato sedici " ("DISPLAY"), w623) -> (w625:string)
        n731 = property on="TEMP 2" class="Bool"("DisabledEnum"=w612) -> ()  [unwired: 2 in, 2 out]
        n732 = property on="TEMP1" class="Bool"("DisabledEnum"=w612) -> ()  [unwired: 2 in, 2 out]
        n733 = property on="RANGE UP" class="Bool"("DisabledEnum"=w612) -> ()  [unwired: 2 in, 2 out]
        n734 = property on="EXIT" class="Bool"("DisabledEnum"=w612) -> ()  [unwired: 2 in, 2 out]
        n735 = property on="DCV2" class="Bool"("DisabledEnum"=w612) -> ()  [unwired: 2 in, 2 out]
        n736 = property on="DCV1" class="Bool"("DisabledEnum"=w612) -> ()  [unwired: 2 in, 2 out]
        n737 = property on="RANGE DOWN" class="Bool"("DisabledEnum"=w612) -> ()  [unwired: 2 in, 2 out]
        n738 = local write "DISPLAY"(w625) -> ()
        n739 = property on="LEFTARR" class="Bool"("DisabledEnum"=w612) -> ()  [unwired: 2 in, 2 out]
        n740 = property on="RIGHTARR" class="Bool"("DisabledEnum"=w612) -> ()  [unwired: 2 in, 2 out]
      }
      frame 17 {
        w661 = T3."Disabled and Grayed Out" ("Disabled")
        w660 = T3."Enabled" ("Disabled")
        n741 = Unbundle By Name(w664) -> ("Sens"=w658:bool, "Rate"=w659:u16)
        n742 = property on="SCAN" class="Bool"("DisabledEnum"=w661) -> ()  [unwired: 2 in, 2 out]
        n743 = property on="ON/OFF" class="Bool"("DisabledEnum"=w661) -> ()  [unwired: 2 in, 2 out]
        n744 = property on="REL" class="Bool"("DisabledEnum"=w661) -> ()  [unwired: 2 in, 2 out]
        n745 = property on="DIGITS" class="Bool"("DisabledEnum"=w661) -> ()  [unwired: 2 in, 2 out]
        n746 = property on="SAVE" class="Bool"("DisabledEnum"=w661) -> ()  [unwired: 2 in, 2 out]
        n747 = property on="ACAL" class="Bool"("DisabledEnum"=w661) -> ()  [unwired: 2 in, 2 out]
        n748 = property on="SHIFT" class="Bool"("DisabledEnum"=w661) -> ()  [unwired: 2 in, 2 out]
        n749 = property on="V1/V2" class="Bool"("DisabledEnum"=w661) -> ()  [unwired: 2 in, 2 out]
        n750 = property on="STEP" class="Bool"("DisabledEnum"=w661) -> ()  [unwired: 2 in, 2 out]
        n751 = Equal?(x=u16 1, y=w659) -> (x = y?=w673:bool)
        n752 = Equal To 0?(x=w659) -> (x = 0?=w674:bool)
        n753 = Equal?(x=w659, y=u16 2) -> (x = y?=w675:bool)
        n754 = property on="fast 0.1 PLC" class="Str"("Visible"=w673) -> ()  [unwired: 2 in, 2 out]
        n755 = property on="slow 5 PLC" class="Str"("Visible"=w674) -> ()  [unwired: 2 in, 2 out]
        n756 = property on="med 1 PLC" class="Str"("Visible"=w675) -> ()  [unwired: 2 in, 2 out]
        n757 = property on="EX TRIG" class="Bool"("DisabledEnum"=w661) -> ()  [unwired: 2 in, 2 out]
        n758 = property on="TRIG" class="Bool"("DisabledEnum"=w661) -> ()  [unwired: 2 in, 2 out]
        n759 = property on="RECALL" class="Bool"("DisabledEnum"=w661) -> ()  [unwired: 2 in, 2 out]
        n760 = property on="RESTR" class="Bool"("DisabledEnum"=w661) -> ()  [unwired: 2 in, 2 out]
        n761 = property on="VALUE" class="Bool"("DisabledEnum"=w661) -> ()  [unwired: 2 in, 2 out]
        n762 = property on="RATE" class="Bool"("DisabledEnum"=w661) -> ()  [unwired: 2 in, 2 out]
        n763 = property on="AUTO" class="Bool"("DisabledEnum"=w661) -> ()  [unwired: 2 in, 2 out]
        n764 = property on="STORE" class="Bool"("DisabledEnum"=w661) -> ()  [unwired: 2 in, 2 out]
        n765 = property on="FILT" class="Bool"("DisabledEnum"=w661) -> ()  [unwired: 2 in, 2 out]
        n766 = Select(t="internal", s=w658, f="exsternal") -> (s? t:f=w655:string)
        n767 = Concatenate Strings("sens: " ("DISPLAY"), w655) -> (w666:string)
        n768 = local write "DISPLAY"(w666) -> ()
        n769 = property on="ENTER" class="Bool"("DisabledEnum"=w660) -> ()  [unwired: 2 in, 2 out]
        n770 = property on="TEMP 2" class="Bool"("DisabledEnum"=w660) -> ()  [unwired: 2 in, 2 out]
        n771 = property on="TEMP1" class="Bool"("DisabledEnum"=w660) -> ()  [unwired: 2 in, 2 out]
        n772 = property on="RANGE UP" class="Bool"("DisabledEnum"=w660) -> ()  [unwired: 2 in, 2 out]
        n773 = property on="EXIT" class="Bool"("DisabledEnum"=w660) -> ()  [unwired: 2 in, 2 out]
        n774 = property on="DCV2" class="Bool"("DisabledEnum"=w660) -> ()  [unwired: 2 in, 2 out]
        n775 = property on="DCV1" class="Bool"("DisabledEnum"=w660) -> ()  [unwired: 2 in, 2 out]
        n776 = property on="RANGE DOWN" class="Bool"("DisabledEnum"=w660) -> ()  [unwired: 2 in, 2 out]
        n777 = property on="shift" class="Str"("Visible"=w671) -> ()  [unwired: 2 in, 2 out]
        n778 = property on="filt" class="Str"("Visible"=FALSE) -> ()  [unwired: 2 in, 2 out]
        n779 = property on="CH1" class="Str"("Visible"=FALSE) -> ()  [unwired: 2 in, 2 out]
        n780 = property on="AUTO" class="Bool"("Visible"=FALSE) -> ()  [unwired: 2 in, 2 out]
        n781 = property on="CH2" class="Str"("Visible"=FALSE) -> ()  [unwired: 2 in, 2 out]
        n782 = property on="REL" class="Bool"("Visible"=FALSE) -> ()  [unwired: 2 in, 2 out]
        n783 = property on="LEFTARR" class="Bool"("DisabledEnum"=w660) -> ()  [unwired: 2 in, 2 out]
        n784 = property on="RIGHTARR" class="Bool"("DisabledEnum"=w660) -> ()  [unwired: 2 in, 2 out]
        n785 = call "17-tcoupl_sens.vi"("this"=w668, "button"=w670, "settings in"=w664) -> ("next state"=w667:i32, "settings out"=w669:T6)
      }
      frame 18 {
        w692 = T3."Disabled and Grayed Out" ("Disabled")
        w691 = T3."Enabled" ("Disabled")
        n786 = Unbundle By Name(w695) -> ("Sens"=w680:bool, "Rate"=w690:u16)
        n787 = property on="SCAN" class="Bool"("DisabledEnum"=w692) -> ()  [unwired: 2 in, 2 out]
        n788 = property on="ON/OFF" class="Bool"("DisabledEnum"=w692) -> ()  [unwired: 2 in, 2 out]
        n789 = property on="REL" class="Bool"("DisabledEnum"=w692) -> ()  [unwired: 2 in, 2 out]
        n790 = property on="DIGITS" class="Bool"("DisabledEnum"=w692) -> ()  [unwired: 2 in, 2 out]
        n791 = property on="SAVE" class="Bool"("DisabledEnum"=w692) -> ()  [unwired: 2 in, 2 out]
        n792 = property on="ACAL" class="Bool"("DisabledEnum"=w692) -> ()  [unwired: 2 in, 2 out]
        n793 = property on="SHIFT" class="Bool"("DisabledEnum"=w692) -> ()  [unwired: 2 in, 2 out]
        n794 = property on="V1/V2" class="Bool"("DisabledEnum"=w692) -> ()  [unwired: 2 in, 2 out]
        n795 = property on="STEP" class="Bool"("DisabledEnum"=w692) -> ()  [unwired: 2 in, 2 out]
        n796 = Equal?(x=u16 1, y=w690) -> (x = y?=w704:bool)
        n797 = Equal To 0?(x=w690) -> (x = 0?=w705:bool)
        n798 = Equal?(x=w690, y=u16 2) -> (x = y?=w706:bool)
        n799 = property on="fast 0.1 PLC" class="Str"("Visible"=w704) -> ()  [unwired: 2 in, 2 out]
        n800 = property on="slow 5 PLC" class="Str"("Visible"=w705) -> ()  [unwired: 2 in, 2 out]
        n801 = property on="med 1 PLC" class="Str"("Visible"=w706) -> ()  [unwired: 2 in, 2 out]
        n802 = Not Equal To 0?(x=w676) -> (x != 0?=w677:bool)
        n803 = Equal?(x=w676, y=-1) -> (x = y?=w679:bool)
        n804 = property on="EX TRIG" class="Bool"("DisabledEnum"=w692) -> ()  [unwired: 2 in, 2 out]
        n805 = Select(t=w680, s=w679, f=w677) -> (s? t:f=w681:bool)
        n806 = property on="TRIG" class="Bool"("DisabledEnum"=w692) -> ()  [unwired: 2 in, 2 out]
        n807 = property on="RECALL" class="Bool"("DisabledEnum"=w692) -> ()  [unwired: 2 in, 2 out]
        n808 = property on="RESTR" class="Bool"("DisabledEnum"=w692) -> ()  [unwired: 2 in, 2 out]
        n809 = property on="VALUE" class="Bool"("DisabledEnum"=w692) -> ()  [unwired: 2 in, 2 out]
        n810 = property on="RATE" class="Bool"("DisabledEnum"=w692) -> ()  [unwired: 2 in, 2 out]
        n811 = property on="AUTO" class="Bool"("DisabledEnum"=w692) -> ()  [unwired: 2 in, 2 out]
        n812 = property on="STORE" class="Bool"("DisabledEnum"=w692) -> ()  [unwired: 2 in, 2 out]
        n813 = property on="FILT" class="Bool"("DisabledEnum"=w692) -> ()  [unwired: 2 in, 2 out]
        n814 = Select(t="internal", s=w681, f="exsternal") -> (s? t:f=w682:string)
        n815 = Concatenate Strings("sens: " ("DISPLAY"), w682) -> (w697:string)
        n816 = local write "DISPLAY"(w697) -> ()
        n817 = property on="ENTER" class="Bool"("DisabledEnum"=w691) -> ()  [unwired: 2 in, 2 out]
        n818 = property on="TEMP 2" class="Bool"("DisabledEnum"=w691) -> ()  [unwired: 2 in, 2 out]
        n819 = property on="TEMP1" class="Bool"("DisabledEnum"=w691) -> ()  [unwired: 2 in, 2 out]
        n820 = property on="RANGE UP" class="Bool"("DisabledEnum"=w691) -> ()  [unwired: 2 in, 2 out]
        n821 = property on="EXIT" class="Bool"("DisabledEnum"=w691) -> ()  [unwired: 2 in, 2 out]
        n822 = property on="DCV2" class="Bool"("DisabledEnum"=w691) -> ()  [unwired: 2 in, 2 out]
        n823 = property on="DCV1" class="Bool"("DisabledEnum"=w691) -> ()  [unwired: 2 in, 2 out]
        n824 = property on="RANGE DOWN" class="Bool"("DisabledEnum"=w691) -> ()  [unwired: 2 in, 2 out]
        n825 = property on="shift" class="Str"("Visible"=w702) -> ()  [unwired: 2 in, 2 out]
        n826 = property on="filt" class="Str"("Visible"=FALSE) -> ()  [unwired: 2 in, 2 out]
        n827 = property on="CH1" class="Str"("Visible"=FALSE) -> ()  [unwired: 2 in, 2 out]
        n828 = property on="AUTO" class="Bool"("Visible"=FALSE) -> ()  [unwired: 2 in, 2 out]
        n829 = property on="CH2" class="Str"("Visible"=FALSE) -> ()  [unwired: 2 in, 2 out]
        n830 = property on="REL" class="Bool"("Visible"=FALSE) -> ()  [unwired: 2 in, 2 out]
        n831 = property on="LEFTARR" class="Bool"("DisabledEnum"=w691) -> ()  [unwired: 2 in, 2 out]
        n832 = property on="RIGHTARR" class="Bool"("DisabledEnum"=w691) -> ()  [unwired: 2 in, 2 out]
        n833 = call "18-tcoupl_sense_bis.vi"("this"=w699, "sens in"=w676, "button"=w701, "settings in"=w695) -> ("next state"=w698:i32, "sens out"=w683:i32, "settings out"=w700:T6)
      }
      frame Default {
        w713 = FALSE
        w714 = TRUE
        w712 = T3."Disabled and Grayed Out" ("Disabled")
        w715 = T3."Enabled" ("Disabled")
        n834 = property on="DCV2" class="Bool"("DisabledEnum"=w715) -> ()  [unwired: 2 in, 2 out]
        n835 = property on="RATE" class="Bool"("DisabledEnum"=w712) -> ()  [unwired: 2 in, 2 out]
        n836 = property on="ENTER" class="Bool"("DisabledEnum"=w715) -> ()  [unwired: 2 in, 2 out]
        n837 = property on="AUTO" class="Bool"("DisabledEnum"=w712) -> ()  [unwired: 2 in, 2 out]
        n838 = property on="EXIT" class="Bool"("DisabledEnum"=w715) -> ()  [unwired: 2 in, 2 out]
        n839 = property on="TEMP 2" class="Bool"("DisabledEnum"=w715) -> ()  [unwired: 2 in, 2 out]
        n840 = property on="REL" class="Bool"("DisabledEnum"=w712) -> ()  [unwired: 2 in, 2 out]
        n841 = property on="TEMP1" class="Bool"("DisabledEnum"=w715) -> ()  [unwired: 2 in, 2 out]
        n842 = property on="SCAN" class="Bool"("DisabledEnum"=w712) -> ()  [unwired: 2 in, 2 out]
        n843 = property on="SHIFT" class="Bool"("DisabledEnum"=w712) -> ()  [unwired: 2 in, 2 out]
        n844 = property on="DIGITS" class="Bool"("DisabledEnum"=w712) -> ()  [unwired: 2 in, 2 out]
        n845 = property on="RESTR" class="Bool"("DisabledEnum"=w712) -> ()  [unwired: 2 in, 2 out]
        n846 = property on="V1/V2" class="Bool"("DisabledEnum"=w712) -> ()  [unwired: 2 in, 2 out]
        n847 = property on="RANGE DOWN" class="Bool"("DisabledEnum"=w715) -> ()  [unwired: 2 in, 2 out]
        n848 = property on="ACAL" class="Bool"("DisabledEnum"=w712) -> ()  [unwired: 2 in, 2 out]
        n849 = property on="TRIG" class="Bool"("DisabledEnum"=w712) -> ()  [unwired: 2 in, 2 out]
        n850 = property on="RANGE UP" class="Bool"("DisabledEnum"=w715) -> ()  [unwired: 2 in, 2 out]
        n851 = property on="STEP" class="Bool"("DisabledEnum"=w712) -> ()  [unwired: 2 in, 2 out]
        n852 = property on="FILT" class="Bool"("DisabledEnum"=w712) -> ()  [unwired: 2 in, 2 out]
        n853 = property on="RECALL" class="Bool"("DisabledEnum"=w712) -> ()  [unwired: 2 in, 2 out]
        n854 = property on="VALUE" class="Bool"("DisabledEnum"=w712) -> ()  [unwired: 2 in, 2 out]
        n855 = property on="DCV1" class="Bool"("DisabledEnum"=w715) -> ()  [unwired: 2 in, 2 out]
        n856 = property on="STORE" class="Bool"("DisabledEnum"=w712) -> ()  [unwired: 2 in, 2 out]
        n857 = property on="RIGHTARR" class="Bool"("DisabledEnum"=w715) -> ()  [unwired: 2 in, 2 out]
        n858 = property on="SAVE" class="Bool"("DisabledEnum"=w712) -> ()  [unwired: 2 in, 2 out]
        n859 = property on="EX TRIG" class="Bool"("DisabledEnum"=w712) -> ()  [unwired: 2 in, 2 out]
        n860 = property on="LEFTARR" class="Bool"("DisabledEnum"=w715) -> ()  [unwired: 2 in, 2 out]
        n861 = property on="ON/OFF" class="Bool"("DisabledEnum"=w712) -> ()  [unwired: 2 in, 2 out]
        n862 = local write "DISPLAY"("Default" ("DISPLAY")) -> ()
        n863 = property on="shift" class="Str"("Visible"=w713) -> ()  [unwired: 2 in, 2 out]
        n864 = property on="rel" class="Str"("Visible"=w713) -> ()  [unwired: 2 in, 2 out]
        n865 = property on="CH2" class="Str"("Visible"=w713) -> ()  [unwired: 2 in, 2 out]
        n866 = property on="auto" class="Str"("Visible"=w713) -> ()  [unwired: 2 in, 2 out]
        n867 = property on="med 1 PLC" class="Str"("Visible"=w713) -> ()  [unwired: 2 in, 2 out]
        n868 = property on="slow 5 PLC" class="Str"("Visible"=w714) -> ()  [unwired: 2 in, 2 out]
        n869 = property on="CH1" class="Str"("Visible"=w714) -> ()  [unwired: 2 in, 2 out]
        n870 = property on="fast 0.1 PLC" class="Str"("Visible"=w713) -> ()  [unwired: 2 in, 2 out]
        n871 = property on="filt" class="Str"("Visible"=w713) -> ()  [unwired: 2 in, 2 out]
      }
    }
    n872 = Unbundle By Name(w11) -> ("address"=w10:string)
    n873 = call "RW.vi"("button"=w12, "address string"=w10) -> ("number"=w8:dbl)  [unwired: 1 out]
    n874 = Number To Fractional String(number=w8, precision (6)=i16 8) -> (F-format string=→"DISPLAY":string)  [unwired: 2 in]
    "shift" <- "SHIFT" ("CH2")
    "CH2" <- "CH2" ("CH2")
    "med 1 PLC" <- "MED" ("med 1 PLC")
    "auto" <- "AUTO" ("auto")
    "slow 5 PLC" <- "SLOW" ("slow 5 PLC")
    "fast 0.1 PLC" <- "FAST" ("fast 0.1 PLC")
    "filt" <- "FILT" ("filt")
    "rel" <- "REL" ("rel")
    "CH1" <- "CH1" ("CH1")
  }
